vi "AbelFcsMain.vi"() -> ()   [LabVIEW 2011]
uses:
  <vilib>/vision/Pattern Matching.llb/IMAQ Curve Parameters.ctl
  <vilib>/vision/Pattern Matching.llb/IMAQ Match Range Setting.ctl
  Camera/lib/System Files/user.lib/atmcd32d.llb/Shutter_mode typedef.ctl
  Camera/lib/System Files/user.lib/atmcd32d.llb/Shutter_type typedef.ctl
  <vilib>/vision/Image Controls.llb/IMAQ Rounding Mode.ctl
  Variables/patternImg.vi
  Camera/vi/GlobalSetGetConfigureCamera.vi
  Camera/vi/ccdChipPixels.vi
  Variables/GetPicture.vi
  Variables/GlobalConAxisPI.vi
  Variables/GlobalLaserInterface.vi
  Camera/vi/StopGetPic.vi
  Camera/vi/CamDef.vi
panel:
  out "subarray":dbl[](array[numeric])
  in  "Settings (GeometricMatching)":T3={"Curve Parameters"={"Extraction Mode"=0, "Edge Threshold"=75, "Edge Filter Size"=1, "Min Length"=25, "Row Search Step Size"=15, "Col Search Step Size"=15, "Max Endpoint Gap"=10, "Closed"=FALSE, "Subpixel"=FALSE}, "Match Mode"={"Rotation"=TRUE, "Scale"=FALSE, "Occlusion"=TRUE, "Reserved"=FALSE, "Reserved"=FALSE, "Reserved"=FALSE}, "Range Settings"=[{"Match Constraints"=0, "Min"=0.0, "Max"=360.0}, {"Match Constraints"=2, "Min"=0.0, "Max"=25.0}], "Number of Matches"=5, "Minimum Match Score"=600.0, "SubPixel Accuracy"=FALSE, "Adv. Geometric Match Options 2"=[{"Setup Data Item"=21, "Item Value"=0.0}, {"Setup Data Item"=22, "Item Value"=1.0}]} {"Curve Parameters"."Extraction Mode" items=["Normal", "Uniform Regions"]; "Curve Parameters"."Edge Filter Size" items=["Fine", "Normal", "Contour Tracing"]; "Curve Parameters"."Max Endpoint Gap" min=0; "Curve Parameters"."Col Search Step Size" min=1 max=255 step=1; "Curve Parameters"."Row Search Step Size" min=1 max=255 step=1; "Curve Parameters"."Min Length" min=0; "Curve Parameters"."Edge Threshold" min=1 max=350 step=1; "Range Settings"."Max" format="%.2f"; "Range Settings"."Min" format="%.2f"; "Range Settings"."Match Constraints" items=["Rotation Angle (degrees)", "Scale Factor (%)", "Occlusion (%)"]; "Adv. Geometric Match Options 2"."Setup Data Item" items=["Curve Extraction Mode", "Curve Edge Threshold", "Curve Edge Filter Size", "Min Curve Length", "Curve Row Search Step Size", "Curve Col Search Step Size", "Curve Max Endpoint Gap", "Extract Closed Curves", "Enable Subpixel Curve Extraction", "Enable Correlation Score", "Enable Subpixel Accuracy", "Subpixel Iterations", "Subpixel Tolerance", "Initial Match List Length", "Enable Target Template Curve Score", "Min Match Separation Distance", "Min Match Separation Angle", "Min Match Separation Scale", "Max Match Overlap", "Enable Coarse Result", "Enable Calibration Support", "Enable Contrast Reversal", "Search Strategy", "Refinement Match Factor", "Subpixel Match Factor"]}
  in  "Tab Control":T4(tab)
  out "Histogram":i32[][](graph)
  out "Trace":i32[][](graph)=[[2, 0, 0, 1, 1, 1, 0, 0, 0, 1, 0, 1, 0, 1, 2, 2, 0, 3, 0, 2, 2, 1, 3, 1, 0, 1, 1, 1, 0, 1, 3, 1, 0, 2, 0, 1, 0, 1, 1, 0, 1, 1, 3, 1, 0, 2, 0, 1, 1, 0, 0, 2, 0, 0, 1, 1, 1, 0, 0, 1, 0, 1, 0, 0, 0, 1, 2, 1, 1, 2, 0, 2, 4, 3, 1, 1, 0, 0, 1, 1, 2, 0, 1, 1, 0, 0, 0, 1, 1, 1, 1, 3, 0, 0, 1, 0, 0, 0, 2, 1, 1, 1, 2, 1, 0, 1, 1, 0, 0, 2, 1, 1, 0, 0, 1, 1, 1, 1, 0, 2, 2, 0, 1, 2, 1, 0, 3, 0, 2, 1, 3, 0, 1, 1, 0, 0, 3, 0, 0, 0, 0, 0, 0, 0, 0, 0, 0, 0, 0, 0, 0, 0, 0, 0, 0, 0, 0, 0, 0, 0, 0, 0, 0, 0, 0, 0, 0, 0, 0, 0, 0, 0, 0, 0, 0, 0, 0, 0, 0, 0, 0, 0, 0, 0, 0, 0, 0, 0, 0, 0, 0, 0, 0, 0, 0, 0, 0, 0, 0, 0], [1, 2, 2, 0, 0, 0, 1, 2, 1, 2, 1, 1, 1, 0, 0, 0, 3, 1, 0, 1, 0, 2, 0, 2, 1, 1, 0, 0, 1, 0, 1, 2, 1, 0, 0, 0, 0, 0, 1, 0, 1, 0, 2, 0, 1, 0, 0, 0, 0, 1, 1, 3, 0, 0, 0, 2, 0, 0, 2, 0, 1, 1, 0, 0, 2, 0, 2, 1, 0, 1, 1, 0, 1, 1, 0, 0, 0, 1, 0, 0, 1, 0, 0, 0, 0, 1, 0, 1, 1, 1, 1, 0, 0, 0, 1, 1, 1, 0, 1, 0, 0, 0, 1, 1, 1, 0, 0, 1, 1, 3, 1, 0, 0, 0, 0, 0, 0, 0, 1, 2, 1, 0, 0, 0, 2, 3, 3, 2, 0, 1, 1, 1, 0, 0, 4, 0, 1, 2, 0, 0, 0, 2, 0, 0, 0, 0, 0, 0, 0, 0, 0, 0, 0, 0, 0, 0, 0, 0, 0, 0, 0, 0, 0, 0, 0, 0, 0, 0, 0, 0, 0, 0, 0, 0, 0, 0, 0, 0, 0, 0, 0, 0, 0, 0, 0, 0, 0, 0, 0, 0, 0, 0, 0, 0, 0, 0, 0, 0, 0, 0], [2, 2, 0, 1, 2, 0, 1, 0, 2, 3, 1, 0, 1, 0, 1, 0, 0, 0, 0, 2, 1, 0, 0, 2, 2, 0, 0, 0, 3, 0, 0, 2, 2, 2, 0, 3, 0, 3, 1, 3, 1, 3, 1, 0, 3, 1, 3, 3, 1, 1, 1, 1, 2, 0, 1, 0, 1, 1, 1, 3, 0, 2, 3, 1, 1, 1, 0, 1, 0, 1, 2, 3, 1, 2, 1, 3, 0, 2, 0, 2, 0, 1, 0, 2, 2, 1, 1, 3, 1, 2, 1, 1, 1, 3, 0, 0, 0, 0, 1, 1, 1, 0, 1, 0, 2, 1, 1, 0, 1, 0, 1, 2, 2, 2, 2, 0, 1, 0, 0, 0, 1, 1, 2, 0, 0, 1, 5, 2, 2, 0, 2, 0, 2, 2, 2, 0, 1, 0, 6, 0, 0, 0, 0, 0, 0, 0, 0, 0, 0, 0, 0, 0, 0, 0, 0, 0, 0, 0, 0, 0, 0, 0, 0, 0, 0, 0, 0, 0, 0, 0, 0, 0, 0, 0, 0, 0, 0, 0, 0, 0, 0, 0, 0, 0, 0, 0, 0, 0, 0, 0, 0, 0, 0, 0, 0, 0, 0, 0, 0, 0], [0, 0, 1, 0, 1, 1, 0, 0, 0, 1, 1, 0, 1, 0, 0, 0, 0, 0, 2, 0, 0, 0, 0, 2, 0, 0, 0, 1, 1, 2, 1, 1, 1, 2, 1, 0, 0, 3, 0, 1, 1, 0, 0, 0, 0, 1, 0, 0, 2, 1, 0, 0, 1, 1, 1, 2, 2, 0, 1, 0, 0, 1, 0, 1, 1, 0, 0, 2, 1, 1, 2, 1, 1, 0, 0, 0, 0, 2, 1, 0, 0, 0, 0, 1, 0, 1, 0, 0, 0, 0, 1, 0, 0, 0, 0, 1, 0, 1, 1, 1, 0, 2, 3, 1, 1, 0, 1, 1, 1, 0, 1, 0, 0, 1, 1, 0, 2, 0, 0, 0, 0, 3, 0, 0, 0, 0, 0, 0, 0, 0, 1, 0, 2, 0, 0, 0, 1, 2, 2, 0, 1, 0, 0, 0, 0, 0, 0, 0, 0, 0, 0, 0, 0, 0, 0, 0, 0, 0, 0, 0, 0, 0, 0, 0, 0, 0, 0, 0, 0, 0, 0, 0, 0, 0, 0, 0, 0, 0, 0, 0, 0, 0, 0, 0, 0, 0, 0, 0, 0, 0, 0, 0, 0, 0, 0, 0, 0, 0, 0, 0]]
  out "Point":dbl[][](graph)
  out "Image Out":T5(plugin-control)
  out "Image Number":u32
  out "acquired FPS":dbl
  out "Image":i32[][](graph)
  out "AM image":T5(plugin-control)
  out "Number of Particles":i32
  out "Image 2":dbl[][](graph)
  out "Auto Measure Points":i32
  out "NxtAutMesPoint":i32
  out "Pattern":dbl[][](array[numeric])
  out "X Steps":dbl
  out "3dAbelFcs":bool=TRUE
  out "Y Steps":dbl
  out "Z Steps":dbl
  out "concatenated string":string
  out "Global Stop":bool=TRUE
  out "Stop Measurement":bool
  in  "DeviceTabs":T6(tab)
  in  "WS File Tree":string(tree)
  out "Workspace":path=path "X:/MTusers/Christoph/2011-02-01 Andi/2011-02-01.msw"
  in  "New MSW":bool
  in  "Open MSW":bool
  in  "Sample description":string
  in  "Save Files":bool=TRUE
  out "Last Image File No":i32=-1
  in  "Get Position":bool
  in  "Move Stage":bool
  in  "X-Position":dbl=48.0021 caption="X" min=0.0 max=200.0 step=0.1 format="%1.3f um"
  in  "Y-Position":dbl=19.9997 caption="Y" min=0.0 max=200.0 step=0.1 format="%1.3f um"
  in  "Z-Position":dbl=69.999 caption="Z" min=0.0 max=200.0 step=0.1 format="%1.3f um"
  out "x-position":dbl format="%.3f"
  out "y-position":dbl format="%.3f"
  out "z-position":dbl format="%.3f"
  in  "CFD Settings":T7={"Sync Level"=17, "Sync ZeroX"=0, "Sync Offset"=0, "Chan Settings"=[{"CHx Level"=50, "CHx ZeroX"=10, "CHx Offset"=-22150}, {"CHx Level"=50, "CHx ZeroX"=10, "CHx Offset"=-21850}, {"CHx Level"=75, "CHx ZeroX"=10, "CHx Offset"=-6000}, {"CHx Level"=75, "CHx ZeroX"=10, "CHx Offset"=-5700}]}
  in  "Laser  Profile":string="1"
  in  "Auto Exposure::Mode":u32(ring) items=["Relative"=0, "Ignored"=5]
  in  "Brightness::Mode":u32(ring) items=["Relative"=0, "Ignored"=5]
  in  "Gain::Mode":u32(ring) items=["Absolute"=1, "Auto"=3, "Relative"=0, "Ignored"=5]
  in  "Gamma::Mode":u32(ring)=2 items=["Relative"=0, "Off"=2, "Ignored"=5]
  in  "Shutter::Mode":u32(ring) items=["Auto"=3, "Relative"=0, "Ignored"=5]
  in  "Trigger::Trigger Activation":u32(ring) items=["Level Low", "Level High"]
  in  "Trigger::Trigger Mode":u32(ring)=16 items=["Mode 0"=0, "Mode 1"=1, "Mode 15"=15, "Off"=16]
  in  "Trigger Delay::Mode":u32(ring)=2 items=["Absolute"=1, "Relative"=0, "Off"=2, "Ignored"=5]
  in  "Brightness::Value":dbl=16.0 min=0.0 max=1023.0 step=1.0
  in  "Shutter::Value":dbl=436.0 min=1.0 max=4095.0 step=1.0
  in  "Auto Exposure::Value":dbl=125.0 min=50.0 max=205.0 step=1.0
  in  "Gain::Value":dbl min=0.0 max=680.0 step=1.0
  in  "Trigger::Trigger Parameter":u32 max=0
  in  "Get Temperature":bool
  in  "SET CCD":bool
  in  "OPEN SHUTER":bool
  in  "Close":bool
  in  "Gain":bool
  in  "Start":bool
  in  "Stop":bool
  in  "Exposure":bool
  in  "Set Temperature":bool
  in  "duty cycle":dbl=0.5 format="%.6f"
  in  "frequency":dbl=1.0 format="%.6f"
  in  "PI SystemNumber":i32=1
  in  "Image Measurent Parameters":T8
  in  "Measurement Tab Control":T9(tab)
  in  "SCANNER EMERGENCY":bool
  in  "Stop Program":bool
  out "Task":T10(ring)
  in  "Point Defocussed Cam":bool
  in  "Adjustment":bool
  in  "Laser pulse duration":i32[](array[numeric]) min=2 max=100000 step=1 format="%d µs"
  in  "Measurement Time":i32=60 min=10 format="%.0d s"
  in  "Point Measurement":bool
  out "Counts":u32[](array[numeric])
  in  "Axis":enum32{"x-y", "x-z", "y-x", "y-z", "z-x", "z-y"}(ring)
  in  "Picture size 2":dbl=10.0 min=0.1 max=200.0 format="%1.1f um"
  in  "Picture size":dbl=10.0 min=0.1 max=200.0 format="%1.1f um"
  in  "Pixel time":dbl=3.0 min=0.1 max=100.0 step=0.1 format="%.1f ms"
  in  "Resolution":dbl=0.08 min=0.01 max=10.0 step=0.01 format="%.2f µm"
  out "Measure. time":dbl format="%7.1f s"
  in  "Aquire Image":bool
  out "y":i16=500
  out "x":i16=500
  in  "Save Color Image":bool
  in  "Cam (Defocused)":bool
  in  "How long?":bool
  out "Estimated Time (h)":dbl
  in  "Mesaurement Time (Sec) / Step":dbl
  in  "Start 3D FCS Abel Scan":bool
  in  "FCS Point Measurement":bool
  in  "Z Stepsize":dbl
  in  "Y Stepsize":dbl
  in  "X Stepsize":dbl
  in  "Z End":dbl
  in  "Y End":dbl
  in  "X End":dbl
  in  "Z Start":dbl
  in  "Y Start":dbl
  in  "X Start":dbl
  in  "Find Mols":bool
  in  "Filter":bool=TRUE
  in  "Remove Outliers":i32=10
  in  "Exclude / Include X":bool
  in  "X Start 2":dbl
  in  "X End 2":dbl
  in  "Exclude / Include Y":bool
  in  "Y Start 2":dbl
  in  "Y End 2":dbl
  in  "Measurement Parameter 1":T11 items=["Center of Mass X", "Center of Mass Y", "First Pixel X", "First Pixel Y", "Bounding Rect Left", "Bounding Rect Top", "Bounding Rect Right", "Bounding Rect Bottom", "Max Feret Diameter Start X", "Max Feret Diameter Start Y", "Max Feret Diameter End X", "Max Feret Diameter End Y", "Max Horiz. Segment Length Left", "Max Horiz. Segment Length Right", "Max Horiz. Segment Length Row", "-", "Bounding Rect Width", "Bounding Rect Height", "Bounding Rect Diagonal", "Perimeter", "Convex Hull Perimeter", "Holes' Perimeter", "Max Feret Diameter", "Equivalent Ellipse Major Axis", "Equivalent Ellipse Minor Axis", "Equivalent Ellipse Minor Axis (Feret)", "Equivalent Rect Long Side", "Equivalent Rect Short Side", "Equivalent Rect Diagonal", "Equivalent Rect Short Side (Feret)", "Average Horiz. Segment Length", "Average Vert. Segment Length", "Hydraulic Radius", "Waddel Disk Diameter", "-", "Area", "Holes' Area", "Particle & Holes' Area", "Convex Hull Area", "Image Area", "-", "Number of Holes", "Number of Horiz. Segments", "Number of Vert. Segments", "-", "Orientation", "Max Feret Diameter Orientation", "-", "% Area/Image Area", "% Area/(Particle & Holes' Area)", "Ratio of Equivalent Ellipse Axes", "Ratio of Equivalent Rect Sides", "-", "Elongation Factor", "Compactness Factor", "Heywood Circularity Factor", "Type Factor", "-", "Sum X", "Sum Y", "Sum XX", "Sum XY", "Sum YY", "Sum XXX", "Sum XXY", "Sum XYY", "Sum YYY", "-", "Moment of Inertia XX", "Moment of Inertia XY", "Moment of Inertia YY", "Moment of Inertia XXX", "Moment of Inertia XXY", "Moment of Inertia XYY", "Moment of Inertia YYY", "Norm. Moment of Inertia XX", "Norm. Moment of Inertia XY", "Norm. Moment of Inertia YY", "Norm. Moment of Inertia XXX", "Norm. Moment of Inertia XXY", "Norm. Moment of Inertia XYY", "Norm. Moment of Inertia YYY", "Hu Moment 1", "Hu Moment 2", "Hu Moment 3", "Hu Moment 4", "Hu Moment 5", "Hu Moment 6", "Hu Moment 7"]
  in  "Range Lower Value Par 1":dbl
  in  "Range Upper Value  Par 1":dbl
  in  "Ex/In Par 1":bool
  in  "Measurement Parameter 2":T11 items=["Center of Mass X", "Center of Mass Y", "First Pixel X", "First Pixel Y", "Bounding Rect Left", "Bounding Rect Top", "Bounding Rect Right", "Bounding Rect Bottom", "Max Feret Diameter Start X", "Max Feret Diameter Start Y", "Max Feret Diameter End X", "Max Feret Diameter End Y", "Max Horiz. Segment Length Left", "Max Horiz. Segment Length Right", "Max Horiz. Segment Length Row", "-", "Bounding Rect Width", "Bounding Rect Height", "Bounding Rect Diagonal", "Perimeter", "Convex Hull Perimeter", "Holes' Perimeter", "Max Feret Diameter", "Equivalent Ellipse Major Axis", "Equivalent Ellipse Minor Axis", "Equivalent Ellipse Minor Axis (Feret)", "Equivalent Rect Long Side", "Equivalent Rect Short Side", "Equivalent Rect Diagonal", "Equivalent Rect Short Side (Feret)", "Average Horiz. Segment Length", "Average Vert. Segment Length", "Hydraulic Radius", "Waddel Disk Diameter", "-", "Area", "Holes' Area", "Particle & Holes' Area", "Convex Hull Area", "Image Area", "-", "Number of Holes", "Number of Horiz. Segments", "Number of Vert. Segments", "-", "Orientation", "Max Feret Diameter Orientation", "-", "% Area/Image Area", "% Area/(Particle & Holes' Area)", "Ratio of Equivalent Ellipse Axes", "Ratio of Equivalent Rect Sides", "-", "Elongation Factor", "Compactness Factor", "Heywood Circularity Factor", "Type Factor", "-", "Sum X", "Sum Y", "Sum XX", "Sum XY", "Sum YY", "Sum XXX", "Sum XXY", "Sum XYY", "Sum YYY", "-", "Moment of Inertia XX", "Moment of Inertia XY", "Moment of Inertia YY", "Moment of Inertia XXX", "Moment of Inertia XXY", "Moment of Inertia XYY", "Moment of Inertia YYY", "Norm. Moment of Inertia XX", "Norm. Moment of Inertia XY", "Norm. Moment of Inertia YY", "Norm. Moment of Inertia XXX", "Norm. Moment of Inertia XXY", "Norm. Moment of Inertia XYY", "Norm. Moment of Inertia YYY", "Hu Moment 1", "Hu Moment 2", "Hu Moment 3", "Hu Moment 4", "Hu Moment 5", "Hu Moment 6", "Hu Moment 7"]
  in  "Range Lower Value Par 2":dbl
  in  "Range Upper Value Par 2":dbl
  in  "Ex/In Par 2":bool
  in  "Square/Hexa":bool=TRUE
  in  "Connectivity 4/8":bool
  in  "Manual":bool
  in  "Focuswidth":dbl
  in  "Mode":enum16{"Gauss", "Radial", "Azimuthal"}(ring)
  in  "Detection Modus":u16(ring) items=["Pattern", "Heuristic"]
  in  "NA":dbl
  in  "Auto Defocussed Cam":bool
  in  "Autopoint-Autofocus Z":bool=TRUE
  in  "Auto Measurement Time (ms)":i32=60 caption="Measurement Time (s)" min=10
  out "Auto Meas Progress":i32(slide) caption="Point 34 / 34" scale=0.0..34.0
  in  "Auto Meas":bool
  out "Active pt3":path
  out "Buffer Overrun":bool
  out "Running":bool
  # "Range"
  # "Scanner Position"
  # "Point Measurement Settings"
  # "Start Experiment"
  # "Estimated Mesaurement Time"
  # "Image Scan Settings"
  # "Save as png"
  # "Pixel"
  # "Define the 3D Space and Stepwith of your Experiment"
  # "Time of the Experiment"
  # "Check What to Mesaure"
  # "Start Your Experiment here"
  # "Lifetime Mesaurement Time on each Position"
  # "Define Search Area"
  # "Define Detection Parameters"
  # "Exact Matching"
  # "Operation"
  # "Show Progress"
  # "Automated Mesaurement on Single Molecule Coordinates on the  2D Frame"
  # "Start Your Experiment here"
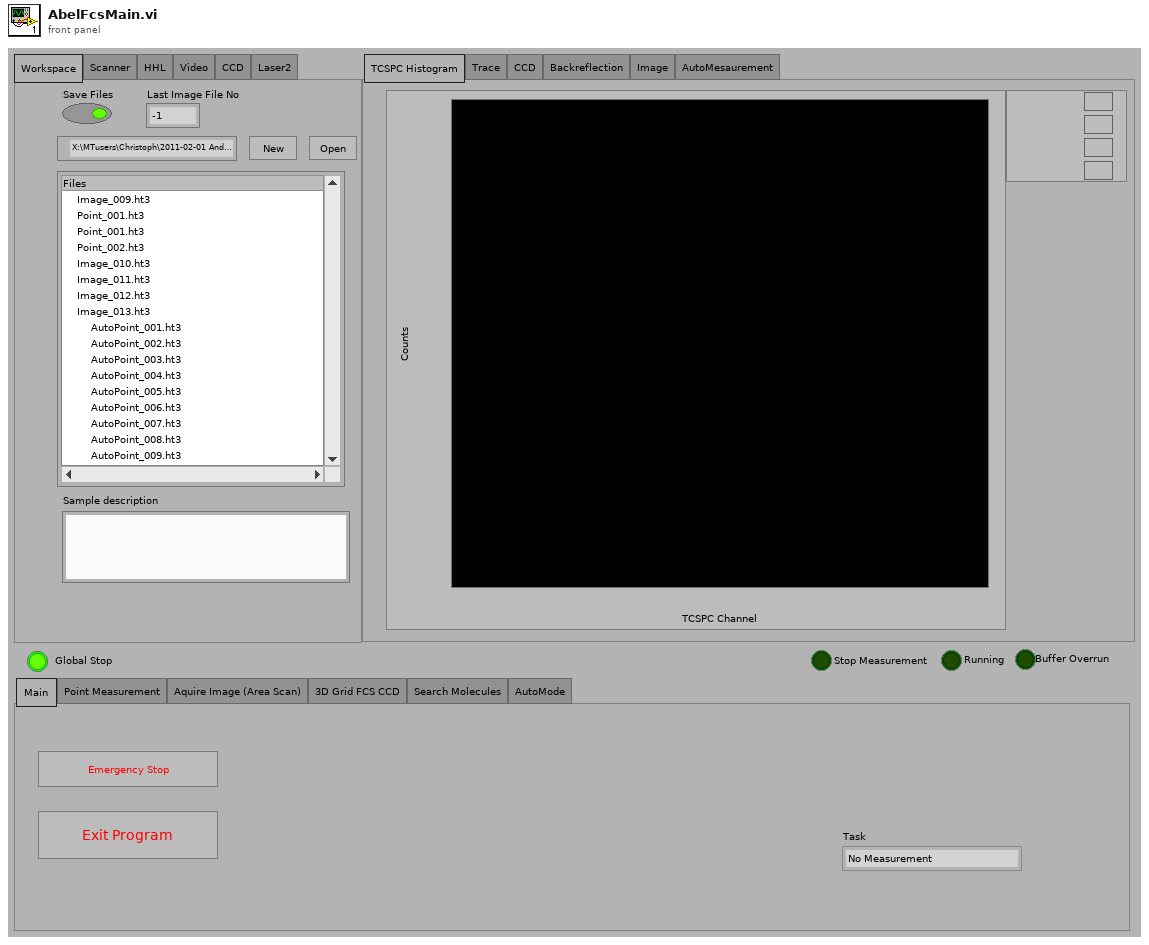
[diagram p1: front panel]
types:
  T1 = typedef "IMAQ Curve Parameters.ctl" = cluster{"Extraction Mode":u32, "Edge Threshold":i32, "Edge Filter Size":u32, "Min Length":i32, "Row Search Step Size":i32, "Col Search Step Size":i32, "Max Endpoint Gap":i32, "Closed":bool, "Subpixel":bool}
  T2 = typedef "IMAQ Match Range Setting.ctl" = cluster{"Match Constraints":u32, "Min":dbl, "Max":dbl}
  T3 = cluster{"Curve Parameters":T1, "Match Mode":cluster{"Rotation":bool, "Scale":bool, "Occlusion":bool, "Reserved":bool, "Reserved":bool, "Reserved":bool}, "Range Settings":T2[], "Number of Matches":i32, "Minimum Match Score":sgl, "SubPixel Accuracy":bool, "Adv. Geometric Match Options 2":cluster{"Setup Data Item":u16, "Item Value":dbl}[]}
  T4 = enum32{"TCSPC Histogram", "Trace", "CCD", "Backreflection", "Image", "AutoMesaurement"}
  T5 = typedef "IMAQ Image.ctl" = refnum<image>
  T6 = enum32{"Workspace", "Scanner", "HHL", "Video", "CCD", "Laser2"}
  T7 = cluster{"Sync Level":i32, "Sync ZeroX":i32, "Sync Offset":i32, "Chan Settings":cluster{"CHx Level":i32, "CHx ZeroX":i32, "CHx Offset":i32}[]}
  T8 = cluster{"Position":cluster{"X-Position":dbl, "Y-Position":dbl, "Z-Position":dbl}, "Axis 1 Pixels":dbl, "Axis 2 Pixels":dbl, "Axis":i32, "Resolution":dbl, "PixelTime":dbl, "Laser pulses":i32}
  T9 = enum32{"Main ", "Point Measurement", "Aquire Image (Area Scan)", "3D Grid FCS CCD", "Search Molecules", "AutoMode"}
  T10 = enum16{"No Measurement", "Aquire Image", "Point Measurement", "Multi Measurement", "Save Color Image", "Find Single Mol.", "Auto Measurement Control", "Auto Point", "Aquire Line Scan", "Grid Measurement", "Trapping", "Move Scanner"}
  T11 = typedef "Particle Parameters" = i32
  T12 = cluster{"Dev":i32, "SerNo":string, "HW_Model":string, "HW_Partno":string}[]
  T13 = enum16{"No Measurement", "Aquire Image", "Point Measurement", "Multi Measurement", "Save Color Image"}
  T14 = enum16{"No Measurement", "Aquire Image", "Point Measurement", "Multi Measurement", "Save Color Image", "Find Single Mol.", "Auto Measurement Control", "Auto Point"}
  T15 = enum16{"No Measurement", "Aquire Image", "Point Measurement", "Multi Measurement", "Save Color Image", "Find Single Mol."}
  T16 = enum16{"Get (Default)", "Set Workspace", "Append File", "Change Comment"}
  T17 = typedef "Shutter_type typedef.ctl" = enum16{"TTL Low", "TTL High"}
  T18 = typedef "Shutter_mode typedef.ctl" = enum16{"Auto", "Open", "Close"}
  T19 = cluster{"File No":i32, "File Path":path, "Parent File":i32, "File Type":enum16{"unknown", "pt3 File", "png Image", "bmp Image"}, "Measurement Type":enum16{"not a pt3 File", "Image File", "Point Measurement", "Auto Point", "Line Scan", "Grid Scan"}, "Upper Left":cluster{"x-Position":dbl, "y-Position":dbl, "z-Position":dbl}, "Pixels":dbl[], "Resolution":dbl, "Scan Axis":enum32{"x-y", "x-z", "y-x", "y-z", "z-x", "z-y"}, "PixelTime":dbl}[]
  T20 = cluster{"File No":i32, "File Path":path, "Parent File":i32, "File Type":enum16{"unknown", "pt3 File", "png Image", "bmp Image"}, "Measurement Type":enum16{"not a pt3 File", "Image File", "Point Measurement", "Auto Point", "Line Scan", "Grid Scan"}, "Upper Left":cluster{"x-Position":dbl, "y-Position":dbl, "z-Position":dbl}, "Pixels":i32[], "Scan Axis":enum32{"x-y", "x-z", "y-x", "y-z", "z-x", "z-y"}, "Resolution":dbl, "PixelTime":dbl}[]
  T21 = cluster{"File No":i32, "File Path":path, "Parent File":i32, "File Type":enum16{"unknown", "pt3 File", "png Image", "bmp Image"}, "Measurement Type":enum16{"not a pt3 File", "Image File", "Point Measurement", "Auto Point", "Line Scan", "Grid Scan"}, "Upper Left":cluster{"x-Position":dbl, "y-Position":dbl, "z-Position":dbl}, "Pixels":i32[], "Resolution":dbl, "Scan Axis":enum32{"x-y", "x-z", "y-z"}, "PixelTime":dbl}[]
  T22 = cluster{"Files in Workspace[0]":cluster{"File No":i32, "File Path":path, "Parent File":i32, "File Type":enum16{"unknown", "pt3 File", "png Image", "bmp Image"}, "Measurement Type":enum16{"not a pt3 File", "Image File", "Point Measurement", "Auto Point", "Line Scan", "Grid Scan"}, "Upper Left":cluster{"x-Position":dbl, "y-Position":dbl, "z-Position":dbl}, "Pixels":i32[], "Scan Axis":enum32{"x-y", "x-z", "y-x", "y-z", "z-x", "z-y"}, "Resolution":dbl, "PixelTime":dbl}, "Files in Workspace[1]":cluster{"File No":i32, "File Path":path, "Parent File":i32, "File Type":enum16{"unknown", "pt3 File", "png Image", "bmp Image"}, "Measurement Type":enum16{"not a pt3 File", "Image File", "Point Measurement", "Auto Point", "Line Scan", "Grid Scan"}, "Upper Left":cluster{"x-Position":dbl, "y-Position":dbl, "z-Position":dbl}, "Pixels":i32[], "Scan Axis":enum32{"x-y", "x-z", "y-x", "y-z", "z-x", "z-y"}, "Resolution":dbl, "PixelTime":dbl}, "Files in Workspace[2]":cluster{"File No":i32, "File Path":path, "Parent File":i32, "File Type":enum16{"unknown", "pt3 File", "png Image", "bmp Image"}, "Measurement Type":enum16{"not a pt3 File", "Image File", "Point Measurement", "Auto Point", "Line Scan", "Grid Scan"}, "Upper Left":cluster{"x-Position":dbl, "y-Position":dbl, "z-Position":dbl}, "Pixels":i32[], "Scan Axis":enum32{"x-y", "x-z", "y-x", "y-z", "z-x", "z-y"}, "Resolution":dbl, "PixelTime":dbl}, "Files in Workspace[3]":cluster{"File No":i32, "File Path":path, "Parent File":i32, "File Type":enum16{"unknown", "pt3 File", "png Image", "bmp Image"}, "Measurement Type":enum16{"not a pt3 File", "Image File", "Point Measurement", "Auto Point", "Line Scan", "Grid Scan"}, "Upper Left":cluster{"x-Position":dbl, "y-Position":dbl, "z-Position":dbl}, "Pixels":i32[], "Scan Axis":enum32{"x-y", "x-z", "y-x", "y-z", "z-x", "z-y"}, "Resolution":dbl, "PixelTime":dbl}, "Files in Workspace[4]":cluster{"File No":i32, "File Path":path, "Parent File":i32, "File Type":enum16{"unknown", "pt3 File", "png Image", "bmp Image"}, "Measurement Type":enum16{"not a pt3 File", "Image File", "Point Measurement", "Auto Point", "Line Scan", "Grid Scan"}, "Upper Left":cluster{"x-Position":dbl, "y-Position":dbl, "z-Position":dbl}, "Pixels":i32[], "Scan Axis":enum32{"x-y", "x-z", "y-x", "y-z", "z-x", "z-y"}, "Resolution":dbl, "PixelTime":dbl}, "Files in Workspace[5]":cluster{"File No":i32, "File Path":path, "Parent File":i32, "File Type":enum16{"unknown", "pt3 File", "png Image", "bmp Image"}, "Measurement Type":enum16{"not a pt3 File", "Image File", "Point Measurement", "Auto Point", "Line Scan", "Grid Scan"}, "Upper Left":cluster{"x-Position":dbl, "y-Position":dbl, "z-Position":dbl}, "Pixels":i32[], "Scan Axis":enum32{"x-y", "x-z", "y-x", "y-z", "z-x", "z-y"}, "Resolution":dbl, "PixelTime":dbl}, "Files in Workspace[6]":cluster{"File No":i32, "File Path":path, "Parent File":i32, "File Type":enum16{"unknown", "pt3 File", "png Image", "bmp Image"}, "Measurement Type":enum16{"not a pt3 File", "Image File", "Point Measurement", "Auto Point", "Line Scan", "Grid Scan"}, "Upper Left":cluster{"x-Position":dbl, "y-Position":dbl, "z-Position":dbl}, "Pixels":i32[], "Scan Axis":enum32{"x-y", "x-z", "y-x", "y-z", "z-x", "z-y"}, "Resolution":dbl, "PixelTime":dbl}, "Files in Workspace[7]":cluster{"File No":i32, "File Path":path, "Parent File":i32, "File Type":enum16{"unknown", "pt3 File", "png Image", "bmp Image"}, "Measurement Type":enum16{"not a pt3 File", "Image File", "Point Measurement", "Auto Point", "Line Scan", "Grid Scan"}, "Upper Left":cluster{"x-Position":dbl, "y-Position":dbl, "z-Position":dbl}, "Pixels":i32[], "Scan Axis":enum32{"x-y", "x-z", "y-x", "y-z", "z-x", "z-y"}, "Resolution":dbl, "PixelTime":dbl}, "Files in Workspace[8]":cluster{"File No":i32, "File Path":path, "Parent File":i32, "File Type":enum16{"unknown", "pt3 File", "png Image", "bmp Image"}, "Measurement Type":enum16{"not a pt3 File", "Image File", "Point Measurement", "Auto Point", "Line Scan", "Grid Scan"}, "Upper Left":cluster{"x-Position":dbl, "y-Position":dbl, "z-Position":dbl}, "Pixels":i32[], "Scan Axis":enum32{"x-y", "x-z", "y-x", "y-z", "z-x", "z-y"}, "Resolution":dbl, "PixelTime":dbl}}
  T23 = typedef "LVPoint32TypeDef.ctl" = cluster{"Horizontal":i32, "Vertical":i32}
  T24 = cluster{"Shift":bool, "Ctrl":bool, "Alt":bool, "Cmd":bool, "Opt":bool}
  T25 = enum16{"No Measurement", "Aquire Image", "Point Measurement", "Multi Measurement", "Save Color Image", "Find Single Mol.", "Auto Measurement Control", "Auto Point", "Aquire Line Scan", "Grid Measurement"}
  T26 = enum16{"none", "fast axis", "slow axis", "both axis", ""}
  T27 = enum16{"none", "fast axis", "slow axis", "both", ""}
  T28 = enum16{"target position", "relative position", "actual position", "position error"}
  T29 = enum16{"not a pt3 File", "Image File", "Point Measurement", "Auto Point"}
  T30 = enum16{"unknown", "pt3 File", "png Image", "bmp Image"}
  T31 = typedef "IMAQ Rounding Mode.ctl" = enum16{"Optimize", "Truncate"}
  T32 = cluster{"Measurement Parameter":T11, "Range Lower Value":dbl, "Range Upper Value":dbl, "Range":bool, "Measurement Type":bool}[]
  T33 = enum16{"not a pt3 File", "Image File", "Point Measurement", "Auto Point", "Line Scan"}
  T34 = cluster{"Dev":i32, "SerNo":string, "HW_Model":string, "HW_Partno":string}
  T35 = cluster{"Comment":string, "Binning":i32, "Offset":i32, "AcquisitionTime (ms)":i32, "HardwareSerial":i32, "SyncDivider":i32, "Resolution (ps)":dbl, "CFD Settings":cluster{"Sync Level":i32, "Sync ZeroX":i32, "Sync Offset":i32, "Chan Settings":cluster{"CHx Level":i32, "CHx ZeroX":i32, "CHx Offset":i32}[]}, "ModuleInfo":cluster{"modelcode":i32, "versioncode":i32}[], "BaseResolution (ps)":dbl, "RefClockSource":i32, "ChanInfo":cluster{"CHx Level":i32, "CHx ZeroX":i32, "CHx Offset":i32, "CHx modidx":i32}[], "SyncRate":i32, "InputsEnabled":i64}
  T36 = cluster{"Dimensions":i32, "Time Per Pixel [ms]":dbl, "Acceleration":i32, "Pattern":i32, "X0":sgl, "Y0":sgl, "Z0":dbl, "PixX":i32, "PixY":i32, "PixResol":sgl, "TStartTo":sgl, "TStoptTo":sgl, "TStartFro":sgl, "TStopFro":sgl}
  T37 = cluster{"InpRateFilePos":i64, "StopAfterFilePos":i64}
  T38 = cluster{"X-Position":dbl, "Y-Position":dbl, "Z-Position":dbl}
  T39 = cluster{"File No":i32, "File Path":path, "Parent File":i32, "File Type":enum16{"unknown", "pt3 File", "png Image", "bmp Image"}, "Measurement Type":enum16{"not a pt3 File", "Image File", "Point Measurement", "Auto Point", "Line Scan", "Grid Scan"}, "Upper Left":cluster{"x-Position":dbl, "y-Position":dbl, "z-Position":dbl}, "Pixels":i32[], "Scan Axis":enum32{"x-y", "x-z", "y-z"}, "Resolution":dbl, "PixelTime":dbl}
  T40 = enum16{"not a pt3 File", "Image File", "Point Measurement", "Auto Point", "Line Scan", "Grid Scan"}
  T41 = cluster{"Ident":string, "Format Version":string, "Creator Name":string, "Creator Version":string, "File Time":string, "Comment":string, "Laser":i32, "Binning":i32, "Offset":i32, "AcquisitionTime (ms)":i32, "HardwareSerial":i32, "SyncDivider":i32, "Resolution (ps)":dbl, "Rates":dbl[], "SyncRate":dbl, "CFD Settings":cluster{"Sync Level":i32, "Sync ZeroX":i32, "Sync Offset":i32, "Chan Settings":cluster{"CHx Level":i32, "CHx ZeroX":i32, "CHx Offset":i32}[]}}
  T42 = cluster{"x-Position":dbl, "y-Position":dbl, "z-Position":dbl}
  T43 = typedef "Image Type" = u32
  T44 = cluster{"MesaurementSelection[0]":cluster{"Measurement Parameter":T11, "Range Lower Value":dbl, "Range Upper Value":dbl, "Range":bool, "Measurement Type":bool}, "MesaurementSelection[1]":cluster{"Measurement Parameter":T11, "Range Lower Value":dbl, "Range Upper Value":dbl, "Range":bool, "Measurement Type":bool}, "MesaurementSelection[2]":cluster{"Measurement Parameter":T11, "Range Lower Value":dbl, "Range Upper Value":dbl, "Range":bool, "Measurement Type":bool}, "MesaurementSelection[3]":cluster{"Measurement Parameter":T11, "Range Lower Value":dbl, "Range Upper Value":dbl, "Range":bool, "Measurement Type":bool}, "MesaurementSelection[4]":cluster{"Measurement Parameter":T11, "Range Lower Value":dbl, "Range Upper Value":dbl, "Range":bool, "Measurement Type":bool}, "MesaurementSelection[5]":cluster{"Measurement Parameter":T11, "Range Lower Value":dbl, "Range Upper Value":dbl, "Range":bool, "Measurement Type":bool}, "MesaurementSelection[6]":cluster{"Measurement Parameter":T11, "Range Lower Value":dbl, "Range Upper Value":dbl, "Range":bool, "Measurement Type":bool}, "MesaurementSelection[7]":cluster{"Measurement Parameter":T11, "Range Lower Value":dbl, "Range Upper Value":dbl, "Range":bool, "Measurement Type":bool}, "MesaurementSelection[8]":cluster{"Measurement Parameter":T11, "Range Lower Value":dbl, "Range Upper Value":dbl, "Range":bool, "Measurement Type":bool}}
  T45 = cluster{"Measurement Parameter":T11, "Range Lower Value":dbl, "Range Upper Value":dbl, "Range":bool, "Measurement Type":bool}
  T46 = typedef "IMAQ Point" = cluster{"X":sgl, "Y":sgl}
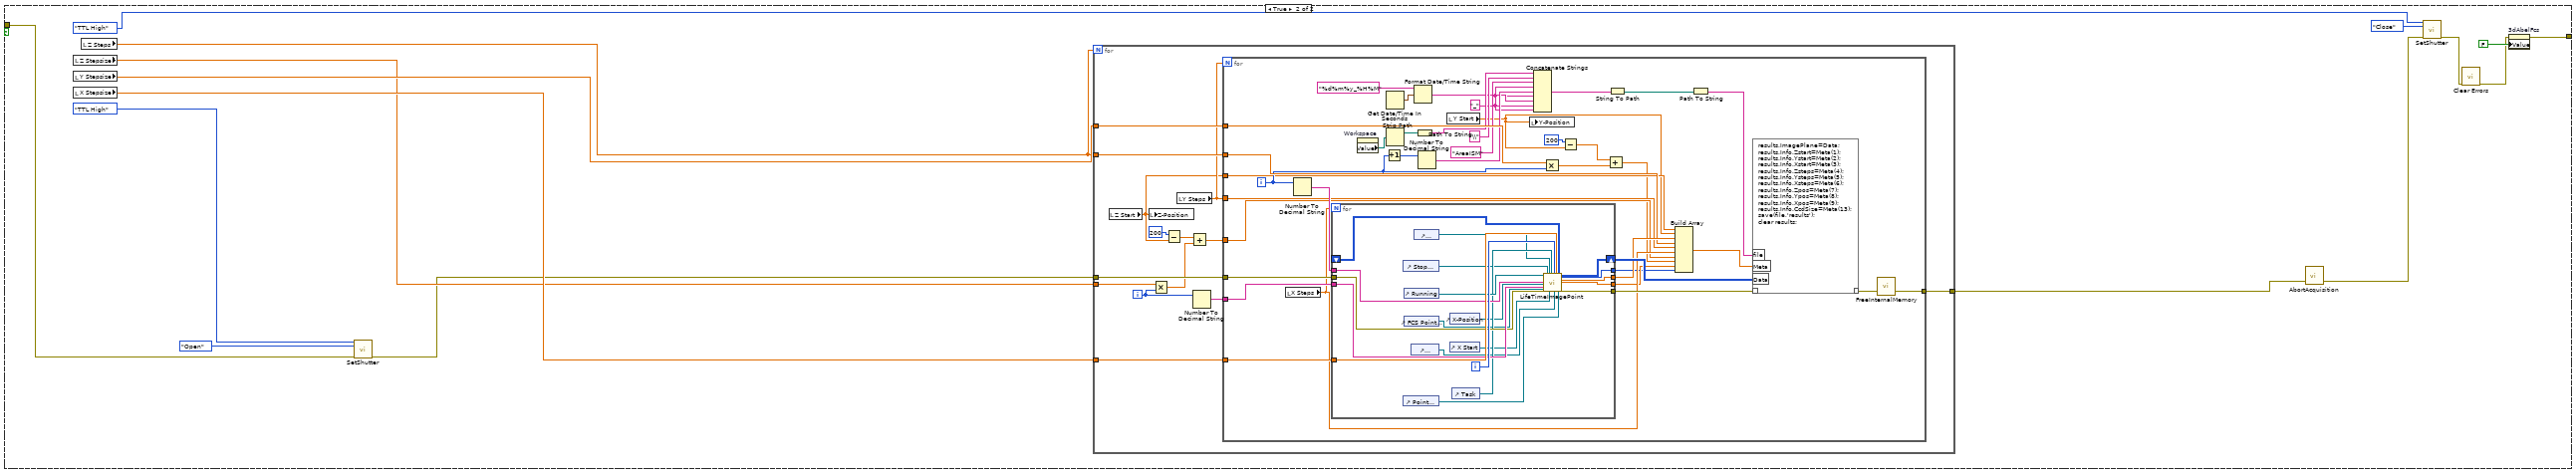
[diagram p2: hidden frame]
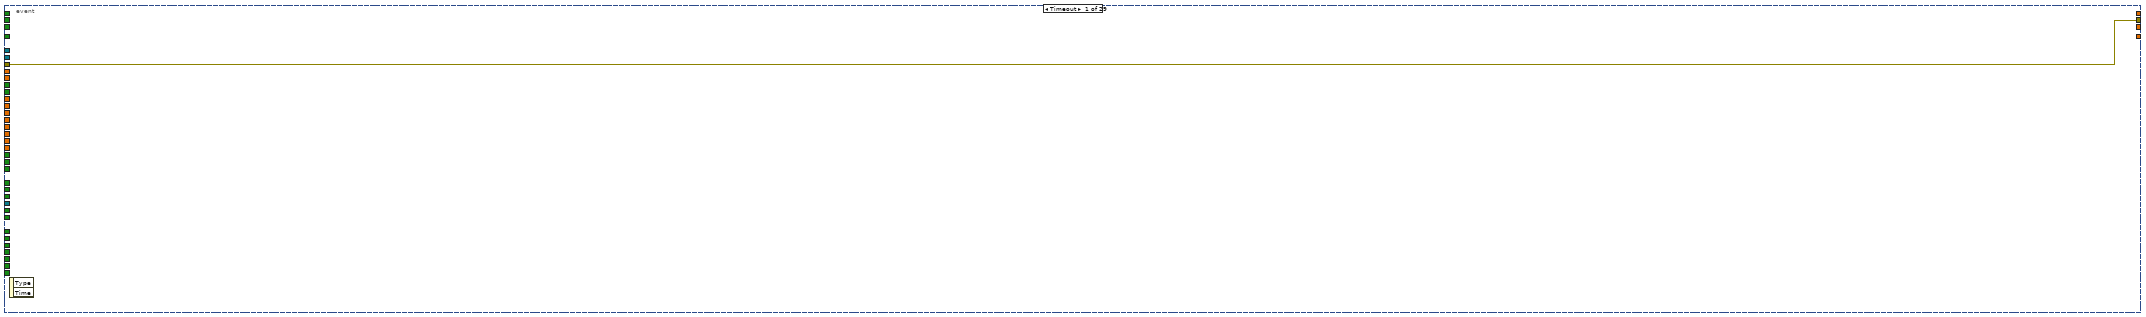
[diagram p3: hidden frame]
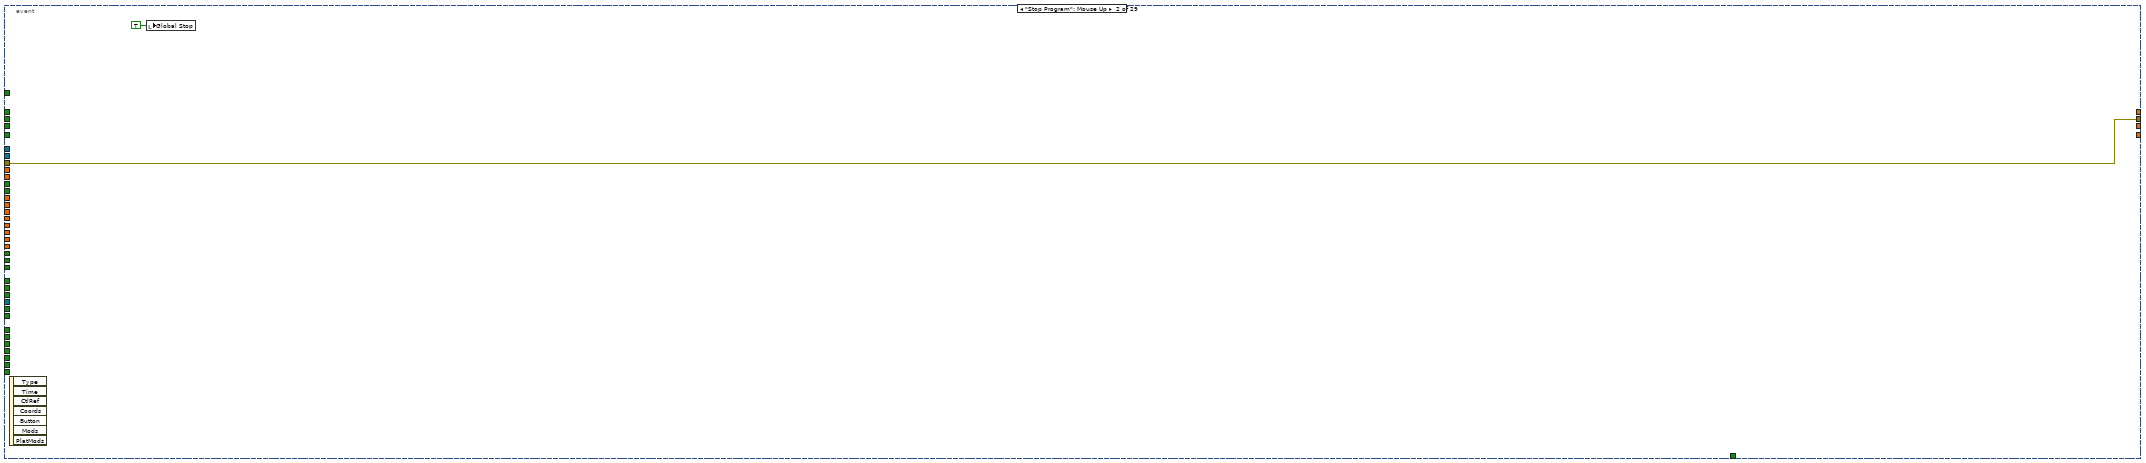
[diagram p4: hidden frame]
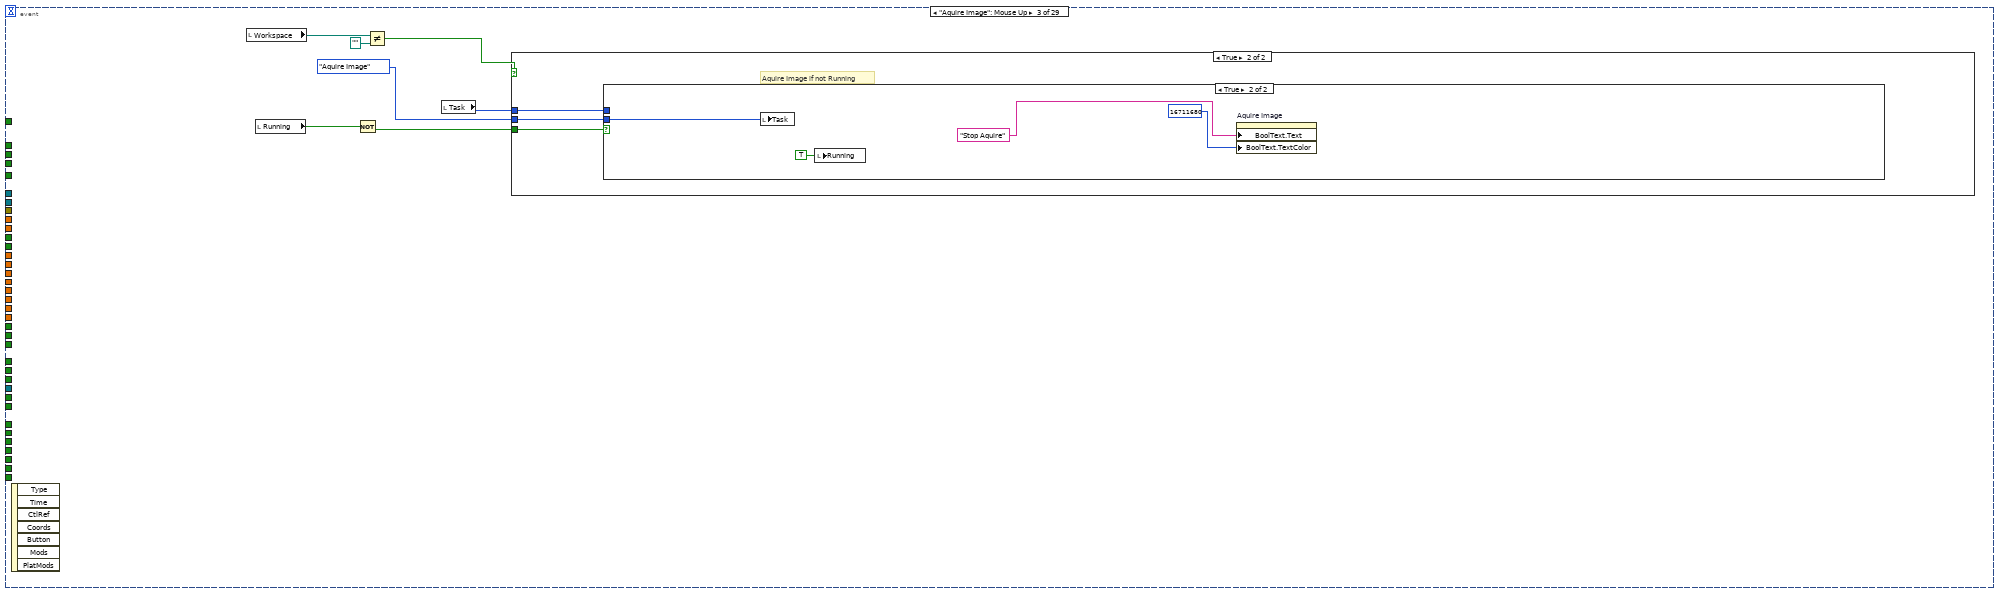
[diagram p5: hidden frame]
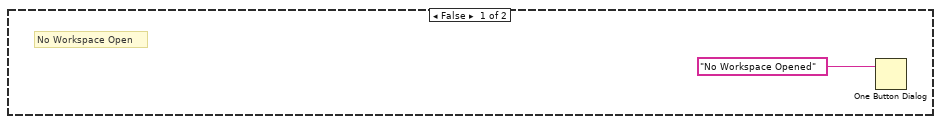
[diagram p6: hidden frame]
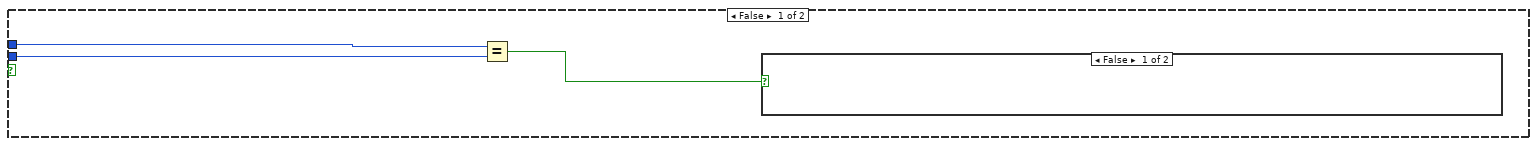
[diagram p7: hidden frame]
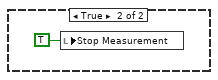
[diagram p8: hidden frame]
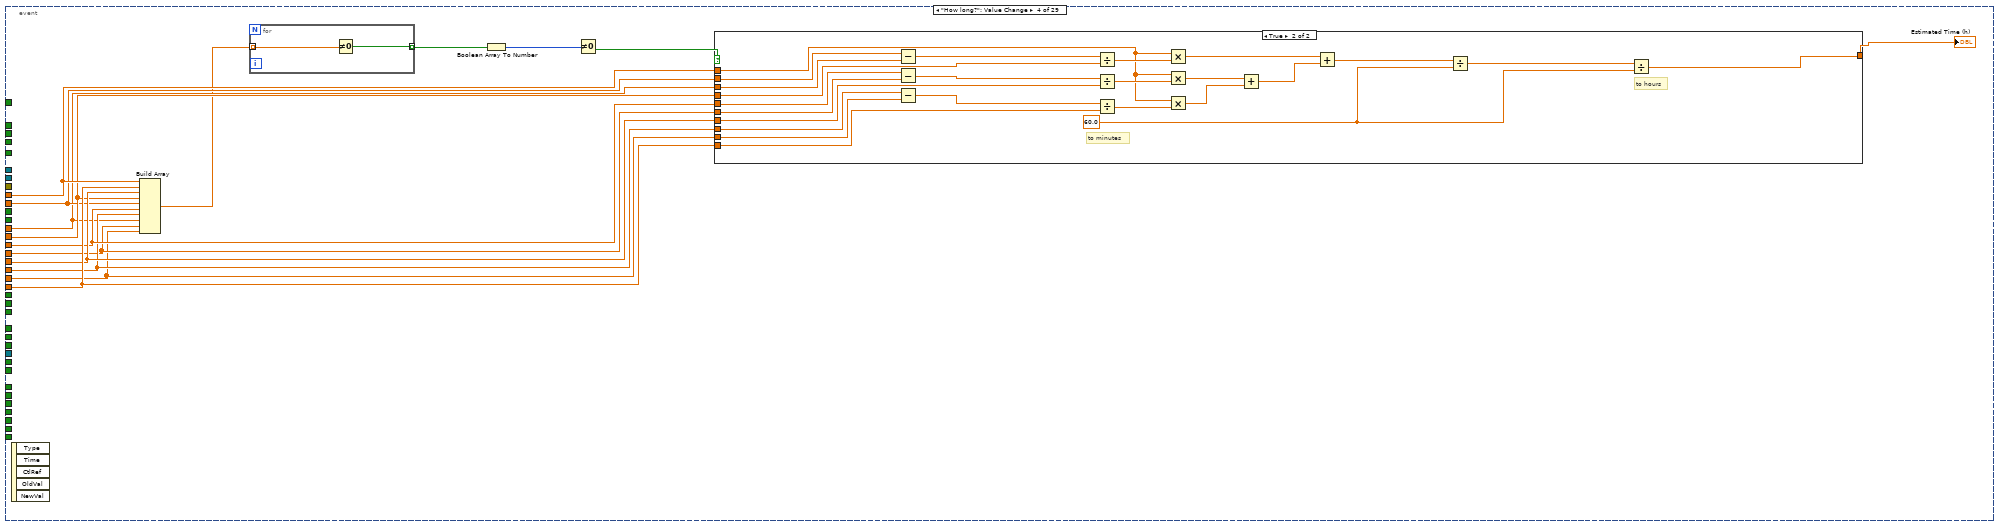
[diagram p9: hidden frame]
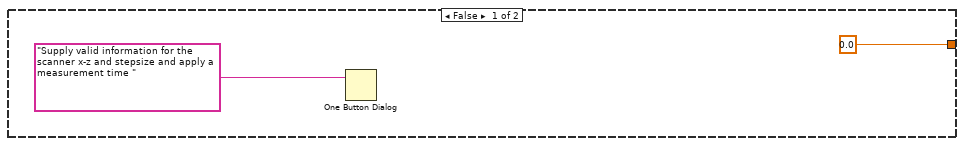
[diagram p10: hidden frame]
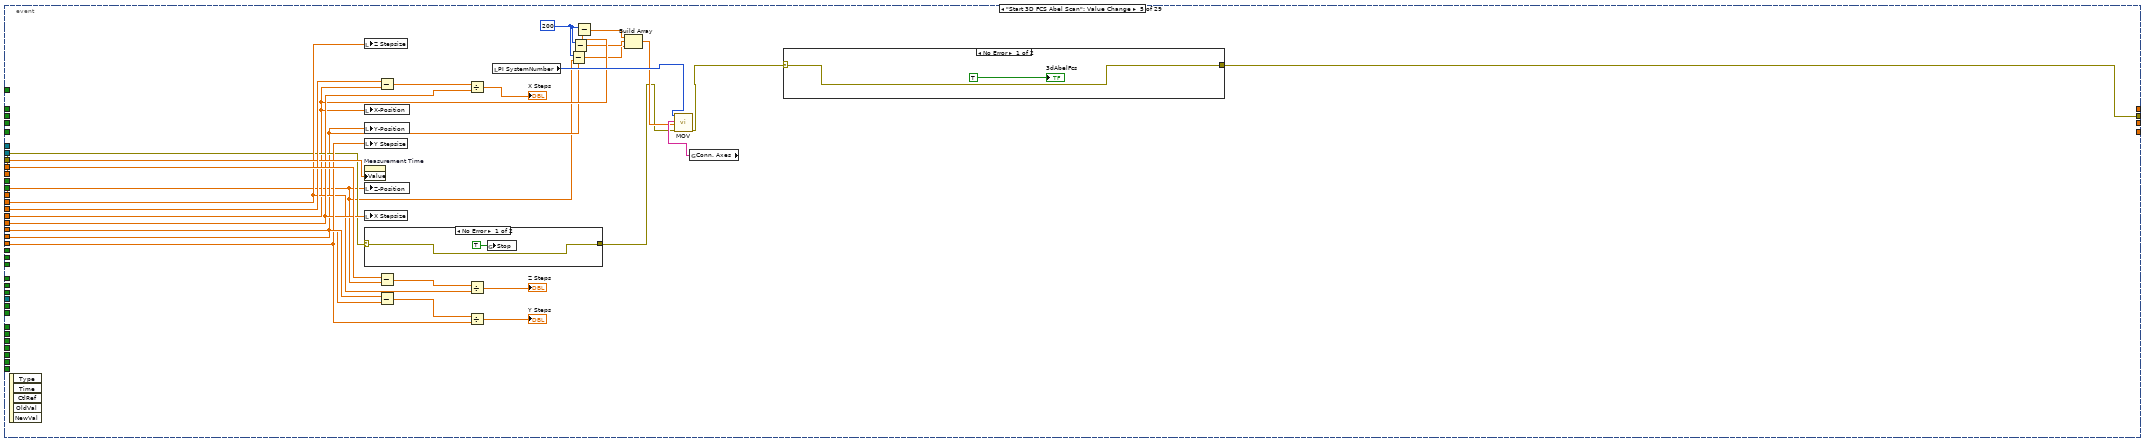
[diagram p11: hidden frame]
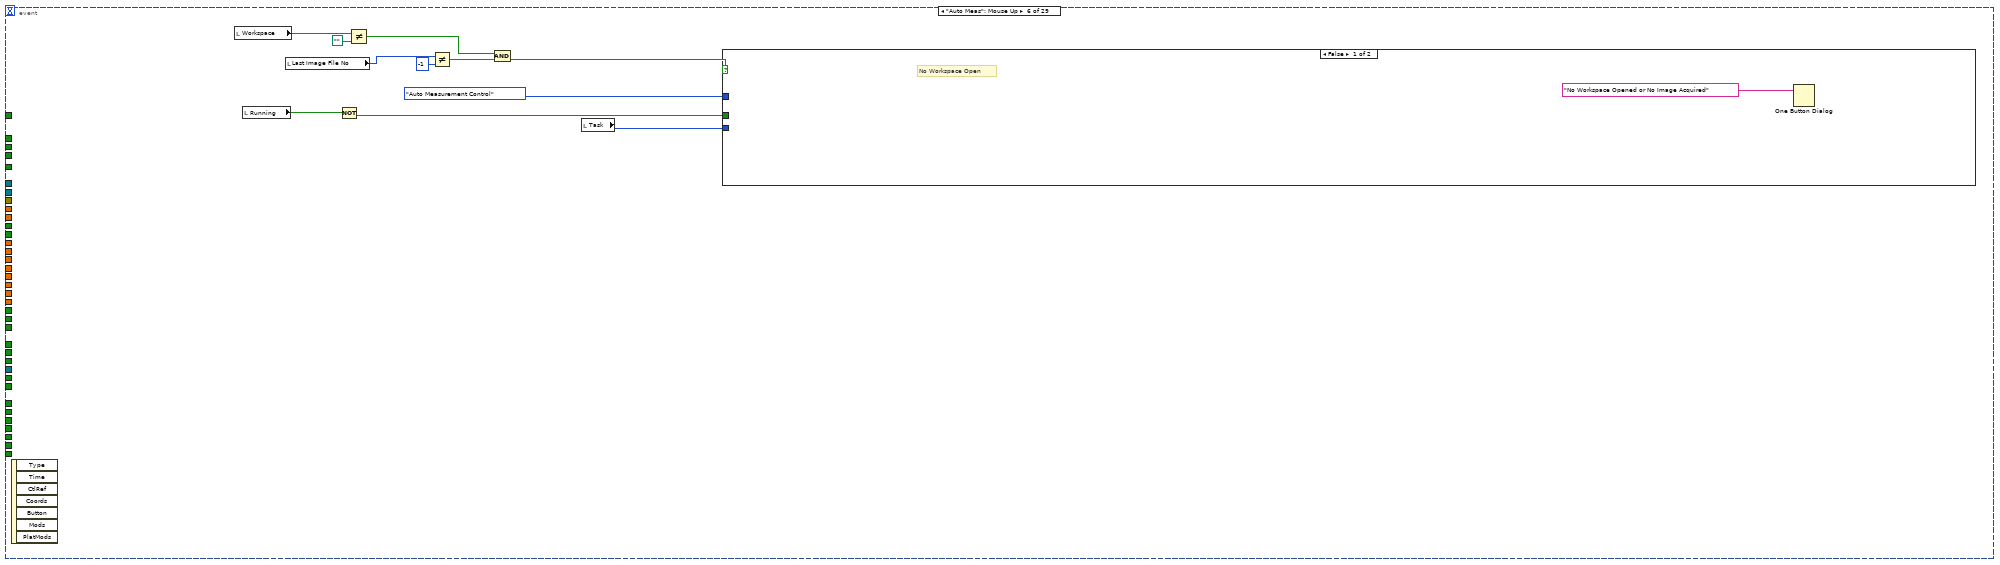
[diagram p14: hidden frame]
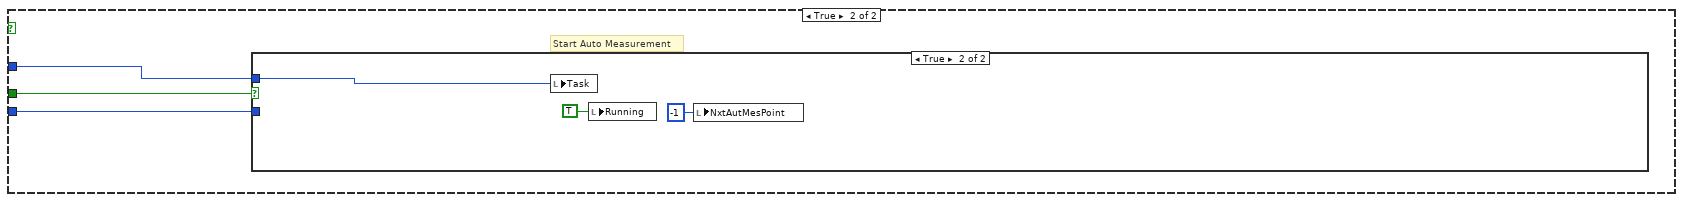
[diagram p15: hidden frame]
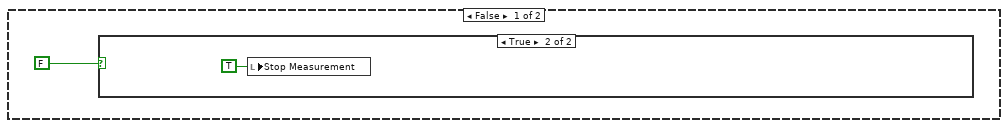
[diagram p16: hidden frame]
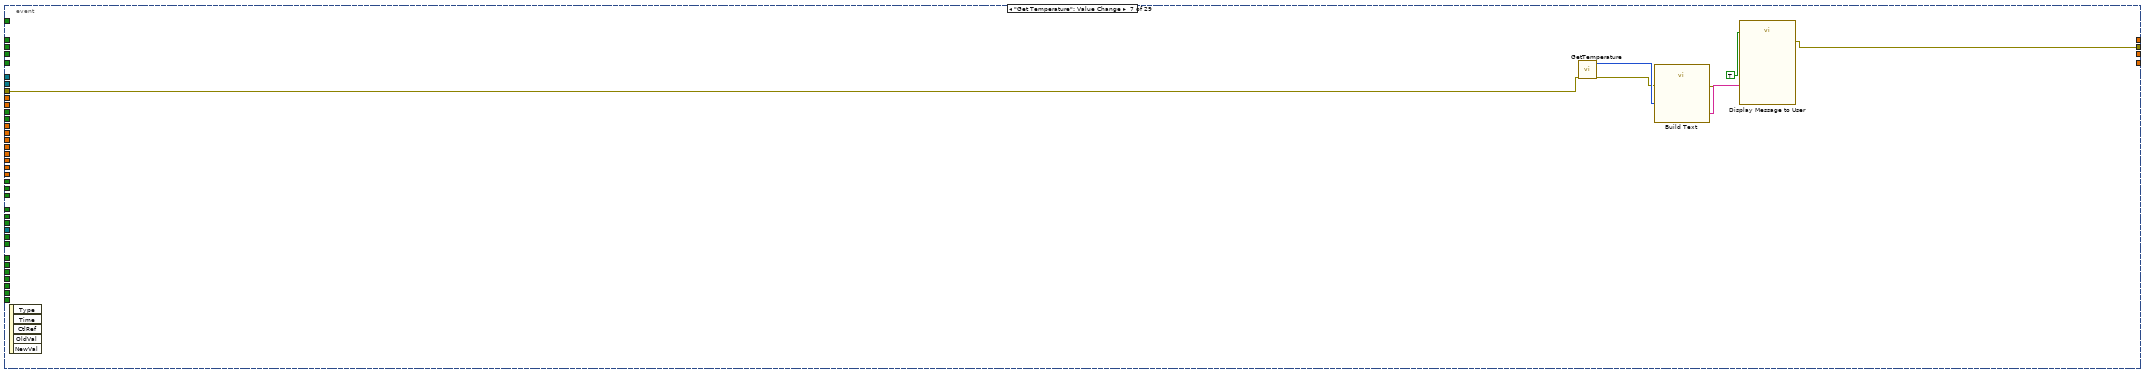
[diagram p18: hidden frame]
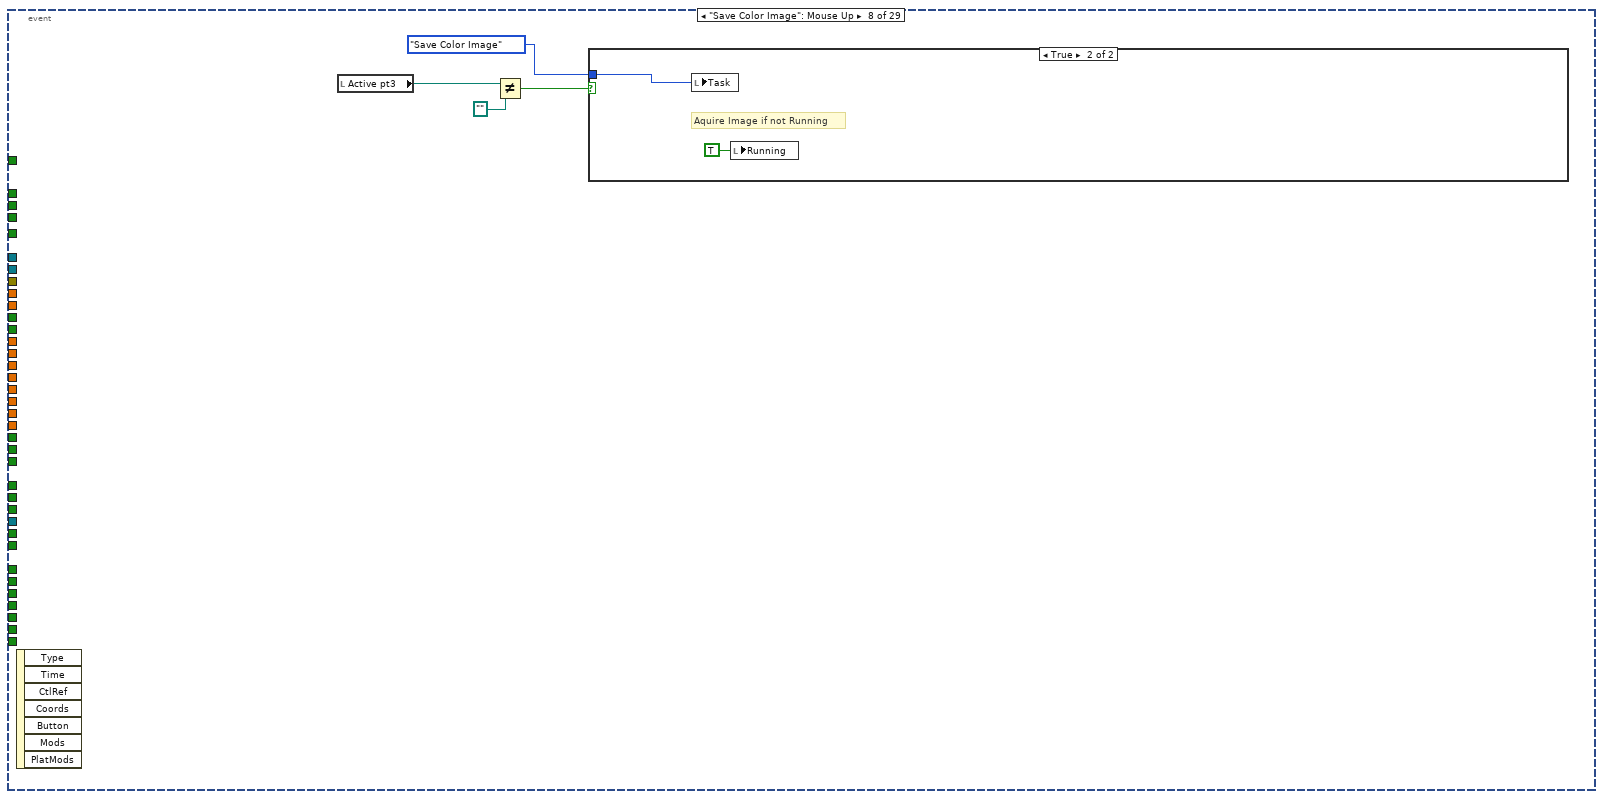
[diagram p19: hidden frame]
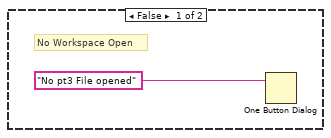
[diagram p20: hidden frame]
diagram:
  n1 = flat-sequence {
    tunnel: [w20] -> w14
    tunnel: errorcluster {"status"=FALSE, "code"=0, "source"=""} ("error in") -> [w31]
    frame #0 {
      (unwired) 1.0 ("CCD Chip Vertical Start")
      w32 = path ""
      w39 = FALSE ("Global Stop")
      n2 = control-ref of="WS File Tree"() -> (w38:refnum<vi>)
      n3 = global write "GetPicture.vi" "GetPicture"(FALSE ("GetPicture")) -> ()
      n4 = local write "Last Image File No"(-1 ("Last Image File No")) -> ()
      n5 = global write "GlobalSetGetConfigureCamera.vi" "gain"(30 ("gain")) -> ()
      n6 = global write "GlobalSetGetConfigureCamera.vi" "Exposure"(sgl 0.1 ("Exposure")) -> ()
      n7 = flat-sequence {
        tunnel: 1.0 ("Vertical Binning") -> [w45]
        tunnel: 1.0 ("CCD Chip Horizontal Start") -> [w44]
        tunnel: 1.0 ("CCD Chip Vertical Start") -> [w40]
        tunnel: 10.0 ("CCD Chip Horizontal End") -> [w43]
        tunnel: 100.0 ("CCD Chip Vertical End") -> [w42]
        tunnel: 1.0 ("Horizontal Binning") -> [w41]
        frame #0 {
          n8 = global write "GlobalSetGetConfigureCamera.vi" "Hbin"(w41) -> ()
          n9 = global write "GlobalSetGetConfigureCamera.vi" "Vbin"(w44) -> ()
          n10 = global write "GlobalSetGetConfigureCamera.vi" "Vbin"(w45) -> ()
          n11 = Subtract(x=w43, y=w44) -> (x-y=w47:dbl)
          n12 = Subtract(x=w42, y=w40) -> (x-y=w46:dbl)
          n13 = global write "ccdChipPixels.vi" "CCD Chip Vertical end"(w42) -> ()
          n14 = global write "ccdChipPixels.vi" "CCD Chip Vertical Start"(w40) -> ()
          n15 = global write "ccdChipPixels.vi" "CCD Chip horizontal end"(w43) -> ()
          n16 = global write "ccdChipPixels.vi" "CCD Chip horizontal start"(w40) -> ()
          n17 = Increment(x=w47) -> (x+1=w49:dbl)
          n18 = Increment(x=w46) -> (x+1=w48:dbl)
          n19 = Multiply(x=w49, y=w48) -> (x*y=w50:dbl)
          n20 = global write "ccdChipPixels.vi" "CCD Chip Size"(w50) -> ()
        }
      }
      n21 = property on="Aquire Image" class="Bool"("BoolText.Text"="Aquire Image" ("Caption.Text"), "BoolText.TextColor"=u32 0 ("Boolean Text.Colors:FG Color")) -> ()  [unwired: 2 in, 2 out]
      n22 = local write "PI SystemNumber"(1 ("PI SystemNumber")) -> ()
      n23 = property on="Point Measurement" class="Bool"("BoolText.Text"="Point Measurement" ("Caption.Text"), "BoolText.TextColor"=u32 0 ("Boolean Text.Colors:FG Color")) -> ()  [unwired: 2 in, 2 out]
      n24 = call "MTS_ClearWSTree2.vi"("error in"=w31, "Tree Refnum"=w38) -> ("error out"=w20:errorcluster)  [unwired: 8 in, 1 out]
      "Global Stop" <- w39
      "Running" <- w39
      "Buffer Overrun" <- w39
      "Stop Measurement" <- w39
      "Workspace" <- w32
      "Active pt3" <- w32
      "Task" <- T10."No Measurement" ("Do Measurement")
    }
  }
  n25 = local read "PI SystemNumber"() -> (w9:i32)
  n26 = control-ref of="X-Position"() -> (w13:refnum<vi>)
  n27 = control-ref of="Y-Position"() -> (w12:refnum<vi>)
  n28 = control-ref of="Z-Position"() -> (w11:refnum<vi>)
  n29 = call "AndorPhysikInstrumenteInitialisiation.vi"("reference"=w13, "error in (no error)"=w14, "reference 3"=w11, "reference 2"=w12, "Pi"=w9) -> ("error out"=w6:errorcluster, "Device List"=w18:T12)  [unwired: 5 in]
  n30 = while {
    shift-right: [w54] -> _
    shift-left: w6 -> [w55]
    stop <- w52 stop-if-true
    n31 = Wait (ms)(milliseconds to wait=u32 100) -> ()  [unwired: 1 out]
    n32 = local read "Global Stop"() -> (w52:bool)
    n33 = control-ref of="Point"() -> (w51:refnum<vi>)
    n34 = call "RunCameraPreview.vi"("error in (no error)"=w55, "Point 2"=w51) -> ("error out"=w54:errorcluster)  [unwired: 9 in]
  }
  n35 = while {
    tunnel: w6 -> [w72]
    stop <- w58 stop-if-true
    n36 = local read "Global Stop"() -> (w73:bool)
    n37 = local read "Global Stop"() -> (w58:bool)
    n38 = call "Vision Acquisition"("Auto Exposure::Mode"="Auto Exposure::Mode", "Auto Exposure::Value"="Auto Exposure::Value", "Brightness::Mode"="Brightness::Mode", "Brightness::Value"="Brightness::Value", "Gain::Mode"="Gain::Mode", "Stop (F)"=w73, "Gain::Value"="Gain::Value", "error in"=w72, "Gamma::Mode"="Gamma::Mode", "Shutter::Mode"="Shutter::Mode", "Shutter::Value"="Shutter::Value", "Trigger::Trigger Activation"="Trigger::Trigger Activation", "Trigger::Trigger Mode"="Trigger::Trigger Mode", "Trigger::Trigger Parameter"="Trigger::Trigger Parameter", "Trigger Delay::Mode"="Trigger Delay::Mode") -> ("Image Out"=→"Image Out":T5, "Image Number"=→"Image Number":u32, "Frame Rate"=→"acquired FPS":dbl)  [unwired: 8 in, 2 out]
  }
  n39 = while {
    shift-right: [w113] -> _
    shift-left: w6 -> [w115]
    stop <- w114 stop-if-true
    n40 = local read "Global Stop"() -> (w114:bool)
    n41 = control-ref of="WS File Tree"() -> (w88:refnum<vi>)
    n42 = global read "GlobalLaserInterface.vi" "InterfaceLaserInitalised"() -> (w76:refnum<visa-resource-name>)
    n43 = event shown="[10] \"X-Position\", \"Y-Position\", \"Z-Position\": Value Change;  \"Move Stage\": Mouse Up" {
      selector: _ -> [_ _ _ _ _ _ _ _ _ _ _ _ _ _ _ _ _ _ _ _ _ _ _ _ _ _ _ _ _]
      dyn-events: _ -> [_ _ _ _ _ _ _ _ _ _ _ _ _ _ _ _ _ _ _ _ _ _ _ _ _ _ _ _ _]
      timeout: _ -> [_ _ _ _ _ _ _ _ _ _ _ _ _ _ _ _ _ _ _ _ _ _ _ _ _ _ _ _ _]
      tunnel: w115 -> [w116 w118 _ _ w193 _ w236 _ _ _ w279 w332 w335 w371 _ w431 _ w471 w478 w507 _ w517 w526 w537 w539 _ _ _ w546]
      tunnel: [w116 w118 _ _ w194 _ w235 _ _ _ w278 w324 w333 w368 _ w430 _ w470 _ _ _ w515 _ w536 _ _ _ _ w547] -> w113
      tunnel: w88 -> [_ _ _ _ _ _ _ _ _ _ _ _ w337 w372 _ _ _ _ _ _ _ _ _ _ _ _ _ _ _]
      tunnel: "Aquire Image" -> [_ _ _ _ _ _ _ _ _ _ _ _ _ _ _ _ _ _ _ _ _ _ _ _ _ _ _ _ _]
      tunnel: "Save Color Image" -> [_ _ _ _ _ _ _ _ _ _ _ _ _ _ _ _ _ _ _ _ _ _ _ _ _ _ _ _ _]
      tunnel: "Open MSW" -> [_ _ _ _ _ _ _ _ _ _ _ _ _ _ _ _ _ _ _ _ _ _ _ _ _ _ _ _ _]
      tunnel: "Find Mols" -> [_ _ _ _ _ _ _ _ _ _ _ _ _ _ _ _ _ _ _ _ _ _ _ _ _ _ _ _ _]
      tunnel: "Auto Meas" -> [_ _ _ _ _ _ _ _ _ _ _ _ _ _ _ _ _ _ _ _ _ _ _ _ _ _ _ _ _]
      tunnel: "New MSW" -> [_ _ _ _ _ _ _ _ _ _ _ _ _ _ _ _ _ _ _ _ _ _ _ _ _ _ _ _ _]
      tunnel: "Stop Program" -> [_ _ _ _ _ _ _ _ _ _ _ _ _ _ _ _ _ _ _ _ _ _ _ _ _ _ _ _ _]
      tunnel: "Point Measurement" -> [_ _ _ _ _ _ _ _ _ _ _ _ _ _ _ _ _ _ _ _ _ _ _ _ _ _ _ _ _]
      tunnel: "Move Stage" -> [_ _ _ _ _ _ _ _ _ _ _ _ _ _ _ _ _ _ _ _ _ _ _ _ _ _ _ _ _]
      tunnel: w76 -> [_ _ _ _ _ _ _ _ _ _ _ _ _ _ _ _ _ _ _ _ _ _ _ _ _ _ _ _ _]
      tunnel: "Get Position" -> [_ _ _ _ _ _ _ _ _ _ _ _ _ _ _ _ _ _ _ _ _ _ _ _ _ _ _ _ _]
      tunnel: [_ _ _ _ _ _ _ _ _ _ w274 w317 _ _ _ _ _ _ _ _ _ _ _ _ _ _ _ _ _] -> w103
      tunnel: [_ _ _ _ _ _ _ _ _ _ w275 w318 _ _ _ _ _ _ _ _ _ _ _ _ _ _ _ _ _] -> w87
      tunnel: [_ _ _ _ _ _ _ _ _ _ w276 w319 _ _ _ _ _ _ _ _ _ _ _ _ _ _ _ _ _] -> w102
      tunnel: "How long?" -> [_ _ _ _ _ _ _ _ _ _ _ _ _ _ _ _ _ _ _ _ _ _ _ _ _ _ _ _ _]
      tunnel: "Start 3D FCS Abel Scan" -> [_ _ _ _ _ _ _ _ _ _ _ _ _ _ _ _ _ _ _ _ _ _ _ _ _ _ _ _ _]
      tunnel: "Mesaurement Time (Sec) / Step" -> [_ _ _ w152 w198 _ _ _ _ _ _ _ _ _ _ _ _ _ _ _ _ _ _ _ _ _ w544 _ _]
      tunnel: "Y Stepsize" -> [_ _ _ w151 w197 _ _ _ _ _ _ _ _ _ _ _ _ _ _ _ _ _ _ _ _ _ _ _ _]
      tunnel: "X Stepsize" -> [_ _ _ w150 w196 _ _ _ _ _ _ _ _ _ _ _ _ _ _ _ _ _ _ _ _ _ _ _ _]
      tunnel: "Z Stepsize" -> [_ _ _ w149 w195 _ _ _ _ _ _ _ _ _ _ _ _ _ _ _ _ _ _ _ _ _ _ _ _]
      tunnel: "FCS Point Measurement" -> [_ _ _ _ _ _ _ _ _ _ _ _ _ _ _ _ _ _ _ _ _ _ _ _ _ _ _ _ _]
      tunnel: "Z End" -> [_ _ _ w148 w207 _ _ _ _ _ _ _ _ _ _ _ _ _ _ _ _ _ _ _ _ _ _ _ _]
      tunnel: "X End" -> [_ _ _ w147 w201 _ _ _ _ _ _ _ _ _ _ _ _ _ _ _ _ _ _ _ _ _ _ _ _]
      tunnel: "Y End" -> [_ _ _ w146 w204 _ _ _ _ _ _ _ _ _ _ _ _ _ _ _ _ _ _ _ _ _ _ _ _]
      tunnel: "Z Start" -> [_ _ _ w145 w187 _ _ _ _ _ _ _ _ _ _ _ _ _ _ _ _ _ _ _ _ _ _ _ _]
      tunnel: "X Start" -> [_ _ _ w144 w189 _ _ _ _ _ _ _ _ _ _ _ _ _ _ _ _ _ _ _ _ _ _ _ _]
      tunnel: "Y Start" -> [_ _ _ w143 w188 _ _ _ _ _ _ _ _ _ _ _ _ _ _ _ _ _ _ _ _ _ _ _ _]
      tunnel: w88 -> [_ _ _ _ _ _ _ _ _ _ _ _ _ _ _ _ _ _ _ _ _ _ _ _ _ _ _ _ _]
      tunnel: "SET CCD" -> [_ _ _ _ _ _ _ _ _ _ _ _ _ _ _ _ _ _ _ _ _ _ _ _ _ _ _ _ _]
      tunnel: "OPEN SHUTER" -> [_ _ _ _ _ _ _ _ _ _ _ _ _ _ _ _ _ _ _ _ _ w516 _ _ _ _ _ _ _]
      tunnel: "Close" -> [_ _ _ _ _ _ _ _ _ _ _ _ _ _ _ _ _ _ _ _ _ _ w525 _ _ _ _ _ _]
      tunnel: "Stop" -> [_ _ _ _ _ _ _ _ _ _ _ _ _ _ _ _ _ _ _ _ _ _ _ _ _ _ _ _ _]
      tunnel: "Start" -> [_ _ _ _ _ _ _ _ _ _ _ _ _ _ _ _ _ _ _ _ _ _ _ _ _ _ _ _ _]
      tunnel: "Gain" -> [_ _ _ _ _ _ _ _ _ _ _ _ _ _ _ _ _ _ _ _ _ _ _ _ _ _ _ _ _]
      tunnel: "Cam (Defocused)" -> [_ _ _ _ _ _ _ _ _ _ _ _ _ _ _ _ _ _ _ _ w514 _ _ _ _ _ _ _ _]
      tunnel: "Set Temperature" -> [_ _ _ _ _ _ _ _ _ _ _ _ _ _ _ _ _ _ _ _ _ _ _ _ _ _ _ _ _]
      tunnel: "SCANNER EMERGENCY" -> [_ _ _ _ _ _ _ _ _ _ _ _ _ _ _ _ _ _ _ _ _ _ _ _ _ _ _ _ _]
      tunnel: "Get Temperature" -> [_ _ _ _ _ _ _ _ _ _ _ _ _ _ _ _ _ _ _ _ _ _ _ _ _ _ _ _ _]
      event Timeout {
        n44 = event-data() -> ()  [unwired: 1 in, 2 out]
      }
      event "Stop Program": Mouse Up {
        n45 = event-data() -> ()  [unwired: 1 in, 7 out]
        n46 = local write "Global Stop"(TRUE ("Global Stop")) -> ()
      }
      event "Aquire Image": Mouse Up {
        n47 = event-data() -> ()  [unwired: 1 in, 7 out]
        n48 = local read "Workspace"() -> (w122:path)
        n49 = local read "Running"() -> (w125:bool)
        n50 = Not(x=w125) -> (.not. x?=w124:bool)
        n51 = Not Equal?(x=w122, y=path "") -> (x != y?=w120:bool)
        n52 = local read "Task"() -> (w119:T10)
        n53 = case shown="True" w120 {
          tunnel: w124 -> [_ w129]
          tunnel: T13."Aquire Image" ("Do Measurement") -> [_ w128]
          tunnel: w119 -> [_ w127]
          frame False {
            # "No Workspace Open"
            n54 = One Button Dialog(message="No Workspace Opened") -> ()  [unwired: 1 in, 1 out]
          }
          frame True {
            # "Aquire Image if not Running"
            n55 = case shown="True" w129 {
              tunnel: w128 -> [w132 w135]
              tunnel: w127 -> [w130 _]
              frame False {
                n56 = Equal?(x=w130, y=w132) -> (x = y?=w131:bool)
                n57 = case shown="False" w131 {
                  frame False {
                  }
                  frame True {
                    n58 = local write "Stop Measurement"(TRUE ("Stop Measurement")) -> ()
                  }
                }
              }
              frame True {
                n59 = local write "Task"(w135) -> ()
                n60 = local write "Running"(TRUE ("Measurement Running")) -> ()
                n61 = property on="Aquire Image" class="Bool"("BoolText.Text"="Stop Aquire" ("Caption.Text"), "BoolText.TextColor"=u32 16711680 ("Boolean Text.Colors:FG Color")) -> ()  [unwired: 2 in, 2 out]
              }
            }
          }
        }
      }
      event "How long?": Value Change {
        n62 = event-data() -> ()  [unwired: 1 in, 5 out]
        n63 = Build Array(w152, w151, w150, w149, w148, w147, w146, w145, w144, w143) -> (w142:dbl[])
        n64 = for {
          tunnel: w142 -> [w180] mode=indexing
          tunnel: [w179] -> w141 mode=indexing
          n65 = Not Equal To 0?(x=w180) -> (x != 0?=w179:bool)
        }
        n66 = Boolean Array To Number(Boolean array=w141) -> (number=w140:u32)
        n67 = Not Equal To 0?(x=w140) -> (x != 0?=w139:bool)
        n68 = case shown="True" w139 {
          tunnel: [0.0 w165] -> w138
          tunnel: w152 -> [_ w164]
          tunnel: w151 -> [_ w163]
          tunnel: w150 -> [_ w162]
          tunnel: w149 -> [_ w161]
          tunnel: w148 -> [_ w160]
          tunnel: w147 -> [_ w159]
          tunnel: w146 -> [_ w158]
          tunnel: w145 -> [_ w157]
          tunnel: w144 -> [_ w156]
          tunnel: w143 -> [_ w155]
          frame False {
            n69 = One Button Dialog(message="Supply valid information for the scanner x-z and stepsize and apply a measurement time ") -> ()  [unwired: 1 in, 1 out]
          }
          frame True {
            w166 = 60.0 ("y")
            # "to hours"
            # "to minutes"
            n70 = Subtract(x=w160, y=w157) -> (x-y=w173:dbl)
            n71 = Subtract(x=w159, y=w156) -> (x-y=w178:dbl)
            n72 = Subtract(x=w158, y=w155) -> (x-y=w175:dbl)
            n73 = Divide(x=w173, y=w161) -> (x/y=w174:dbl)
            n74 = Divide(x=w178, y=w162) -> (x/y=w177:dbl)
            n75 = Divide(x=w175, y=w163) -> (x/y=w176:dbl)
            n76 = Multiply(x=w164, y=w174) -> (x*y=w170:dbl)
            n77 = Multiply(x=w164, y=w177) -> (x*y=w172:dbl)
            n78 = Multiply(x=w164, y=w176) -> (x*y=w171:dbl)
            n79 = Add(x=w172, y=w171) -> (x+y=w169:dbl)
            n80 = Add(x=w170, y=w169) -> (x+y=w168:dbl)
            n81 = Divide(x=w168, y=w166) -> (x/y=w167:dbl)
            n82 = Divide(x=w167, y=w166) -> (x/y=w165:dbl)
          }
        }
        "Estimated Time (h)" <- w138
      }
      event "Start 3D FCS Abel Scan": Value Change {
        w190 = 200
        n83 = event-data() -> ()  [unwired: 1 in, 5 out]
        n84 = local write "Z Stepsize"(w195) -> ()
        n85 = local write "X-Position"(w189) -> ()
        n86 = local write "Y-Position"(w188) -> ()
        n87 = local write "Y Stepsize"(w197) -> ()
        n88 = property on="Measurement Time" class="DigNum (strict)"("Value"=w198) -> ()  [unwired: 2 in, 2 out]
        n89 = local write "Z-Position"(w187) -> ()
        n90 = local write "X Stepsize"(w196) -> ()
        n91 = case shown="No Error" w193 {
          selector: w193 -> [w208 w210]
          tunnel: [w208 w210] -> w182
          frame No Error {
            n92 = global write "StopGetPic.vi" "Stop"(TRUE ("Stop")) -> ()
          }
          frame Error {
          }
        }
        n93 = Subtract(x=w201, y=w189) -> (x-y=w200:dbl)
        n94 = Subtract(x=w207, y=w187) -> (x-y=w205:dbl)
        n95 = Subtract(x=w204, y=w188) -> (x-y=w203:dbl)
        n96 = Divide(x=w200, y=w196) -> (x/y=→"X Steps":dbl)
        n97 = Divide(x=w205, y=w195) -> (x/y=→"Z Steps":dbl)
        n98 = Divide(x=w203, y=w197) -> (x/y=→"Y Steps":dbl)
        n99 = local read "PI SystemNumber"() -> (w192:i32)
        n100 = Subtract(x=w190, y=w187) -> (x-y=w184:dbl)
        n101 = Subtract(x=w190, y=w188) -> (x-y=w185:dbl)
        n102 = Subtract(x=w190, y=w189) -> (x-y=w186:dbl)
        n103 = Build Array(w186, w185, w184) -> (w183:dbl[])
        n104 = global read "GlobalConAxisPI.vi" "Conn. Axes"() -> (w191:string[])
        n105 = call "MOV.vi"("System no."=w192, "Axes to move"=w191, "Position values"=w183, "error in"=w182) -> ("error out"=w181:errorcluster)  [unwired: 15 in]
        n106 = case shown="No Error" w181 {
          selector: w181 -> [w211 w213]
          tunnel: [w211 w213] -> w194
          frame No Error {
            "3dAbelFcs" <- TRUE
          }
          frame Error {
          }
        }
      }
      event "Auto Meas": Mouse Up {
        n107 = event-data() -> ()  [unwired: 1 in, 7 out]
        n108 = local read "Workspace"() -> (w221:path)
        n109 = local read "Running"() -> (w224:bool)
        n110 = local read "Last Image File No"() -> (w218:i32)
        n111 = Not(x=w224) -> (.not. x?=w223:bool)
        n112 = Not Equal?(x=w221, y=path "") -> (x != y?=w216:bool)
        n113 = Not Equal?(x=w218, y=-1) -> (x != y?=w215:bool)
        n114 = And(x=w216, y=w215) -> (x .and. y?=w214:bool)
        n115 = local read "Task"() -> (w222:T10)
        n116 = case shown="False" w214 {
          tunnel: w223 -> [_ w228]
          tunnel: T14."Auto Measurement Control" ("Do Measurement") -> [_ w227]
          tunnel: w222 -> [_ w226]
          frame False {
            # "No Workspace Open"
            n117 = One Button Dialog(message="No Workspace Opened or No Image Acquired") -> ()  [unwired: 1 in, 1 out]
          }
          frame True {
            # "Start Auto Measurement"
            n118 = case shown="True" w228 {
              tunnel: w227 -> [_ w232]
              tunnel: w226 -> [_ _]
              frame False {
                n119 = case shown="True" FALSE {
                  frame False {
                  }
                  frame True {
                    n120 = local write "Stop Measurement"(TRUE ("Stop Measurement")) -> ()
                  }
                }
              }
              frame True {
                n121 = local write "Task"(w232) -> ()
                n122 = local write "Running"(TRUE ("Measurement Running")) -> ()
                n123 = local write "NxtAutMesPoint"(-1 ("NxtAutMesPoint")) -> ()
              }
            }
          }
        }
      }
      event "Get Temperature": Value Change {
        n124 = event-data() -> ()  [unwired: 1 in, 5 out]
        n125 = call "GetTemperature.vi"("error in (no error)"=w236) -> ("error out"=w237:errorcluster, "temperature"=w240:i32)  [unwired: 3 in, 2 out]
        n126 = call "Build Text"("Cam"=w240, "error in (no error)"=w237) -> ("Result"=w239:string, "error out"=w238:errorcluster)  [unwired: 12 in]
        n127 = call "Display Message to User"("error in (no error)"=w238, "Enable"=TRUE, "Message"=w239) -> ("error out"=w235:errorcluster)  [unwired: 7 in, 1 out]
      }
      event "Save Color Image": Mouse Up {
        n128 = event-data() -> ()  [unwired: 1 in, 7 out]
        n129 = local read "Active pt3"() -> (w243:path)
        n130 = Not Equal?(x=w243, y=path "") -> (x != y?=w241:bool)
        n131 = case shown="True" w241 {
          tunnel: T15."Save Color Image" ("Do Measurement") -> [_ w247]
          frame False {
            # "No Workspace Open"
            n132 = One Button Dialog(message="No pt3 File opened") -> ()  [unwired: 1 in, 1 out]
          }
          frame True {
            # "Aquire Image if not Running"
            n133 = local write "Task"(w247) -> ()
            n134 = local write "Running"(TRUE ("Measurement Running")) -> ()
          }
        }
      }
      event "Find Mols": Mouse Up {
        n135 = event-data() -> ()  [unwired: 1 in, 7 out]
        n136 = local read "Active pt3"() -> (w250:path)
        n137 = Not Equal?(x=w250, y=path "") -> (x != y?=w248:bool)
        n138 = case shown="True" w248 {
          tunnel: T15."Find Single Mol." ("Do Measurement") -> [_ w254]
          frame False {
            # "No Workspace Open"
            n139 = One Button Dialog(message="No pt3 File opened") -> ()  [unwired: 1 in, 1 out]
          }
          frame True {
            # "Aquire Image if not Running"
            n140 = local write "Task"(w254) -> ()
            n141 = local write "Running"(TRUE ("Measurement Running")) -> ()
          }
        }
      }
      event "Point Measurement": Mouse Up {
        n142 = event-data() -> ()  [unwired: 1 in, 7 out]
        n143 = local read "Workspace"() -> (w257:path)
        n144 = local read "Running"() -> (w261:bool)
        n145 = Not(x=w261) -> (.not. x?=w260:bool)
        n146 = Not Equal?(x=w257, y=path "") -> (x != y?=w255:bool)
        n147 = local read "Task"() -> (w258:T10)
        n148 = case shown="True" w255 {
          tunnel: w260 -> [_ w265]
          tunnel: T13."Point Measurement" ("Do Measurement") -> [_ w264]
          tunnel: w258 -> [_ w263]
          frame False {
            # "No Workspace Open"
            n149 = One Button Dialog(message="No Workspace Opened") -> ()  [unwired: 1 in, 1 out]
          }
          frame True {
            # "Aquire Image if not Running"
            n150 = case shown="False" w265 {
              tunnel: w264 -> [w267 w271]
              tunnel: w263 -> [w268 _]
              frame False {
                n151 = Equal?(x=w268, y=w267) -> (x = y?=w266:bool)
                n152 = case shown="False" w266 {
                  frame False {
                  }
                  frame True {
                    n153 = local write "Stop Measurement"(TRUE ("Stop Measurement")) -> ()
                  }
                }
              }
              frame True {
                n154 = local write "Task"(w271) -> ()
                n155 = local write "Running"(TRUE ("Measurement Running")) -> ()
                n156 = property on="Point Measurement" class="Bool"("BoolText.Text"="Stop Aquire" ("Caption.Text"), "BoolText.TextColor"=u32 16711680 ("Boolean Text.Colors:FG Color")) -> ()  [unwired: 2 in, 2 out]
              }
            }
          }
        }
      }
      event "X-Position", "Y-Position", "Z-Position": Value Change; "Move Stage": Mouse Up {
        n157 = event-data() -> ()  [unwired: 1 in, 3 out]
        n158 = local read "Workspace"() -> (w282:path)
        n159 = local read "Running"() -> (w284:bool)
        n160 = local read "PI SystemNumber"() -> (w277:i32)
        n161 = Not(x=w284) -> (.not. x?=w283:bool)
        n162 = Not Equal?(x=w282, y=path "") -> (x != y?=w280:bool)
        n163 = case shown="True" w280 {
          tunnel: w283 -> [_ w292]
          tunnel: w279 -> [_ w291]
          tunnel: [_ w290] -> w278
          tunnel: w277 -> [_ w289]
          tunnel: [_ w288] -> w274
          tunnel: [_ w287] -> w275
          tunnel: [_ w286] -> w276
          frame False {
            # "No Workspace Open"
            n164 = One Button Dialog(message="No Workspace Opened") -> ()  [unwired: 1 in, 1 out]
          }
          frame True {
            # "Move Stage if not Running"
            n165 = case shown="True" w292 {
              tunnel: w291 -> [_ w316]
              tunnel: [_ w306] -> w290
              tunnel: w289 -> [_ w314]
              tunnel: [_ w293] -> w288
              tunnel: [_ w294] -> w287
              tunnel: [_ w295] -> w286
              frame False {
              }
              frame True {
                w298 = 200
                n166 = local read "X-Position"() -> (w301:dbl)
                n167 = local read "Y-Position"() -> (w300:dbl)
                n168 = local read "Z-Position"() -> (w305:dbl)
                n169 = Subtract(x=w298, y=w301) -> (x-y=w302:dbl)
                n170 = Subtract(x=w298, y=w300) -> (x-y=w303:dbl)
                n171 = Subtract(x=w298, y=w305) -> (x-y=w304:dbl)
                n172 = Build Array(w302, w303, w304) -> (w315:dbl[])
                n173 = global read "GlobalConAxisPI.vi" "Conn. Axes"() -> (w313:string[])
                n174 = call "MOV.vi"("System no."=w314, "Axes to move"=w313, "Position values"=w315, "error in"=w316) -> ("error out"=w311:errorcluster)  [unwired: 15 in]
                n175 = call "POS?.vi"("System no."=w314, "Axes to query"=w313, "All axes?"=TRUE, "error in"=w311) -> ("Position"=w310:dbl[], "error out"=w306:errorcluster)  [unwired: 14 in]
                n176 = Index Array(array=w310, index #1=0 ("index"), index #2=1 ("index"), index #3=2 ("index")) -> (element #1=w299:dbl, element #2=w296:dbl, element #3=w297:dbl)
                n177 = Subtract(x=w298, y=w299) -> (x-y=w295:dbl)
                n178 = Subtract(x=w298, y=w296) -> (x-y=w294:dbl)
                n179 = Subtract(x=w298, y=w297) -> (x-y=w293:dbl)
              }
            }
          }
        }
        n180 = property on="y-position" class="DigNum (strict)"("Value"=w275) -> ()  [unwired: 2 in, 2 out]
        n181 = property on="z-position" class="DigNum (strict)"("Value"=w274) -> ()  [unwired: 2 in, 2 out]
        n182 = property on="x-position" class="DigNum (strict)"("Value"=w276) -> ()  [unwired: 2 in, 2 out]
      }
      event "Get Position": Value Change {
        w323 = 200
        n183 = event-data() -> ()  [unwired: 1 in, 5 out]
        n184 = local read "PI SystemNumber"() -> (w331:i32)
        n185 = global read "GlobalConAxisPI.vi" "Conn. Axes"() -> (w330:string[])
        n186 = call "POS?.vi"("System no."=w331, "Axes to query"=w330, "All axes?"=TRUE, "error in"=w332) -> ("Position"=w328:dbl[], "error out"=w324:errorcluster)  [unwired: 14 in]
        n187 = Index Array(array=w328, index #1=0 ("index"), index #2=1 ("index"), index #3=2 ("index")) -> (element #1=w320:dbl, element #2=w321:dbl, element #3=w322:dbl)
        n188 = Subtract(x=w323, y=w320) -> (x-y=w319:dbl)
        n189 = Subtract(x=w323, y=w321) -> (x-y=w318:dbl)
        n190 = Subtract(x=w323, y=w322) -> (x-y=w317:dbl)
        n191 = property on="y-position" class="DigNum (strict)"("Value"=w318) -> ()  [unwired: 2 in, 2 out]
        n192 = property on="x-position" class="DigNum (strict)"("Value"=w319) -> ()  [unwired: 2 in, 2 out]
        n193 = property on="z-position" class="DigNum (strict)"("Value"=w317) -> ()  [unwired: 2 in, 2 out]
      }
      event "New MSW": Mouse Up {
        # "Default Name"
        n194 = event-data() -> ()  [unwired: 1 in, 7 out]
        n195 = flat-sequence {
          tunnel: [w353] -> w336
          tunnel: w335 -> [w353]
          frame #0 {
            n196 = local write "Running"(TRUE ("MeasRunig")) -> ()
          }
        }
        n197 = Get Date/Time In Seconds() -> (seconds since 1Jan1904=w350:timestamp)
        n198 = Format Date/Time String(time format string (%c)="%Y-%m-%d", seconds (now)=w350) -> (date/time string=w348:string)  [unwired: 1 out]
        n199 = Concatenate Strings(w348, ".msw" ("string")) -> (w346:string)
        n200 = call "File Dialog"("start path"=path "D:/", "prompt"="Create New Workspace", "button label"="Create", "default name"=w346, "error in"=w336, "pattern (all files)"="*.msw", "pattern label"="MT Scan Workspace") -> ("selected path"=w340:path, "cancelled"=w341:bool, "error out"=w339:errorcluster)  [unwired: 5 in, 1 out]
        n201 = case shown="False" w341 {
          tunnel: w340 -> [w359 _]
          tunnel: w339 -> [w365 w367]
          tunnel: [w357 w366] -> w334
          tunnel: w337 -> [w355 _]
          frame False {
            # "Create Empty Workspace"
            n202 = local write "Workspace"(w359) -> ()
            n203 = call "MTS_CreateWriteMSW.vi"("Rewrite"=TRUE, "error in (no error)"=w365, "Workspace Path"=w359) -> ("error out"=w358:errorcluster, "Created"=w362:string, "Comment (dup)"=w361:string, "Files in Workspace (dup)"=w360:T19)  [unwired: 5 in]
            n204 = call "MTS_Workspace.vi"("Workspace"=w359, "Operation"=T16."Set Workspace", "Created in"=w362, "New Comment"=w361, "Files in Workspace in"=w360) -> ("Files in Workspace"=w356:T20)  [unwired: 3 in, 3 out]
            n205 = call "MTS_BuildWSTree.vi"("error in"=w358, "Files in Workspace"=w356, "Tree Refnum"=w355) -> ("error out"=w357:errorcluster)  [unwired: 6 in, 2 out]
          }
          frame True {
            n206 = call <vilib>:"Clear Errors.vi"("error in (no error)"=w367) -> ("error out"=w366:errorcluster)  [unwired: 6 in]
          }
        }
        n207 = flat-sequence {
          tunnel: w334 -> [w351]
          tunnel: [w351] -> w333
          frame #0 {
            n208 = local write "Running"(FALSE ("MeasRunig")) -> ()
          }
        }
      }
      event "Open MSW": Mouse Up {
        n209 = event-data() -> ()  [unwired: 1 in, 7 out]
        n210 = flat-sequence {
          tunnel: w371 -> [w383]
          tunnel: [w383] -> w370
          frame #0 {
            n211 = local write "Running"(TRUE ("MeasRunig")) -> ()
          }
        }
        n212 = call "File Dialog2"("start path"=path "D:/", "prompt"="Create New Workspace", "button label"="Open", "error in"=w370, "pattern (all files)"="*.msw", "pattern label"="MT Scan Workspace") -> ("selected path"=w375:path, "cancelled"=w376:bool, "error out"=w374:errorcluster)  [unwired: 6 in, 1 out]
        n213 = case shown="False" w376 {
          tunnel: w375 -> [w391 _]
          tunnel: w374 -> [w396 w398]
          tunnel: [w389 w397] -> w369
          tunnel: w372 -> [w388 _]
          frame False {
            # "Open Workspace"
            n214 = local write "Workspace"(w391) -> ()
            n215 = call "MTS_ReadMSW.vi"("error in (no error)"=w396, "Workspace Path"=w391) -> ("error out"=w390:errorcluster, "Created"=w394:string, "Comment"=w393:string, "Files in Workspace"=w392:T21)  [unwired: 6 in]
            n216 = call "MTS_Workspace.vi"("Workspace"=w391, "Operation"=T16."Set Workspace", "Created in"=w394, "New Comment"=w393, "Files in Workspace in"=w392) -> ("Files in Workspace"=w387:T20)  [unwired: 3 in, 3 out]
            n217 = Array To Cluster(array=w387) -> (cluster=w386:T22)
            n218 = Unbundle By Name(w386) -> ()  [unwired: 1 out]
            n219 = call "MTS_BuildWSTree.vi"("error in"=w390, "Files in Workspace"=w387, "Tree Refnum"=w388) -> ("error out"=w389:errorcluster, "numberOfFilesInWorkspace"=w385:i32)  [unwired: 6 in, 1 out]
            n220 = local write "Last Image File No"(w385) -> ()
          }
          frame True {
            n221 = call <vilib>:"Clear Errors.vi"("error in (no error)"=w398) -> ("error out"=w397:errorcluster)  [unwired: 6 in]
          }
        }
        n222 = flat-sequence {
          tunnel: w369 -> [w381]
          tunnel: [w381] -> w368
          frame #0 {
            n223 = local write "Running"(FALSE ("MeasRunig")) -> ()
          }
        }
      }
      event "Image": Mouse Up {
        w401 = 100.0 ("y")
        n224 = event-data() -> ("Coords"=w413:T23, "PlatMods"=w414:T24)  [unwired: 1 in, 5 out]
        n225 = invoke on="Image" class="IntGraph (strict)" method="Map Coords To XY"("Coords"=w413) -> ("Map Coords To XY"=w410:bool, "XY"=w408:cluster{"X":dbl, "Y":dbl})  [unwired: 6 in, 5 out]
        n226 = Unbundle By Name(w414) -> ("Ctrl"=w411:bool)
        n227 = And(x=w410, y=w411) -> (x .and. y?=w412:bool)
        n228 = Unbundle(w408) -> ("X"=w407:dbl, "Y"=w404:dbl)
        n229 = Multiply(x=w407, y=w401) -> (x*y=w406:dbl)
        n230 = Multiply(x=w404, y=w401) -> (x*y=w403:dbl)
        n231 = Round To Nearest(number=w406) -> (nearest integer value=w405:dbl)
        n232 = Round To Nearest(number=w403) -> (nearest integer value=w402:dbl)
        n233 = Divide(x=w405, y=w401) -> (x/y=w400:dbl)
        n234 = Divide(x=w402, y=w401) -> (x/y=w399:dbl)
        n235 = local read "Axis"() -> (w409:enum32{"x-y", "x-z", "y-x", "y-z", "z-x", "z-y"})
        n236 = case shown="True" w412 {
          tunnel: w409 -> [_ w417]
          tunnel: w400 -> [_ w416]
          tunnel: w399 -> [_ w415]
          frame False {
          }
          frame True {
            n237 = case shown="\"x-y\", Default" w417 {
              tunnel: w416 -> [w419 w421 w423]
              tunnel: w415 -> [w418 w420 w422]
              frame "x-y", Default {
                n238 = local write "X-Position"(w419) -> ()
                n239 = local write "Y-Position"(w418) -> ()
              }
              frame "x-z" {
                n240 = local write "X-Position"(w421) -> ()
                n241 = local write "Z-Position"(w420) -> ()
              }
              frame "y-z" {
                n242 = local write "Y-Position"(w423) -> ()
                n243 = local write "Z-Position"(w422) -> ()
              }
            }
          }
        }
      }
      event "WS File Tree": Value Change {
        n244 = event-data() -> ("NewVal"=w432:string)  [unwired: 1 in, 4 out]
        n245 = control-ref of="Workspace"() -> (w429:refnum<vi>)
        n246 = control-ref of="Histogram"() -> (w427:refnum<vi>)
        n247 = control-ref of="Trace"() -> (w426:refnum<vi>)
        n248 = control-ref of="Image"() -> (w425:refnum<vi>)
        n249 = control-ref of="Image"() -> (w424:refnum<vi>)
        n250 = control-ref of="Active pt3"() -> (w428:refnum<vi>)
        n251 = call "CreateNewWSfile.vi"("reference 5"=w424, "NewVal"=w432, "Image"=w425, "reference in"=w428, "error in (no error)"=w431, "reference 4"=w426, "reference 3"=w427, "Path in"=w429) -> ("error out"=w430:errorcluster)  [unwired: 3 in]
      }
      event "Resolution", "Picture size", "Pixel time", "Picture size 2", "Axis", "Laser  Profile": Value Change {
        n252 = event-data() -> ()  [unwired: 1 in, 5 out]
        n253 = local read "Axis"() -> (w453:enum32{"x-y", "x-z", "y-x", "y-z", "z-x", "z-y"})
        n254 = local read "Picture size"() -> (w455:dbl)
        n255 = local read "X-Position"() -> (w450:dbl)
        n256 = local read "Y-Position"() -> (w449:dbl)
        n257 = local read "Z-Position"() -> (w448:dbl)
        n258 = local read "Resolution"() -> (w447:dbl)
        n259 = local read "Pixel time"() -> (w456:dbl)
        n260 = local write "Axis"(w453) -> ()
        n261 = local read "Picture size 2"() -> (w454:dbl)
        n262 = local read "Laser  Profile"() -> (w437:string)
        n263 = local write "Pixel time"(w456) -> ()
        n264 = call "PI_CheckScan.vi"("Picture size"=w455, "Picture size 2"=w454, "Axis"=w453, "x-Position"=w450, "y-Position"=w449, "z-Position"=w448) -> ("Picture size out"=w451:dbl, "Picture size out 2"=w452:dbl)  [unwired: 8 in, 4 out]
        n265 = String To Byte Array(string=w437) -> (unsigned byte array=w435:u8[])
        n266 = local write "Picture size"(w451) -> ()
        n267 = local write "Picture size 2"(w452) -> ()
        n268 = Divide(x=w451, y=w447) -> (x/y=w459:dbl)
        n269 = Divide(x=w452, y=w447) -> (x/y=w460:dbl)
        n270 = Array Size(array=w435) -> (size(s)=w434:i32)
        n271 = Subtract(x=w435, y=48) -> (x-y=w441:i32[])
        n272 = Round Toward +Infinity(x=w459) -> (ceil(x): smallest int >= x=→"x":dbl)
        n273 = Round Toward +Infinity(x=w460) -> (ceil(x): smallest int >= x=→"y":dbl)
        n274 = Initialize Array(4, w434) -> (w445:i32[])
        n275 = Initialize Array(1, w434) -> (w443:i32[])
        n276 = In Range and Coerce(upper limit=w445, x=w441, lower limit=w443) -> (coerced(x)=w438:i32[])  [unwired: 1 out]
        n277 = Add(x=w438, y=48) -> (x+y=w440:i32[])
        n278 = Byte Array To String(unsigned byte array=w440) -> (string=w436:string)
        n279 = while {
          shift-right: [w465] -> w433
          shift-left: w436 -> [w469]
          i -> [w461]
          stop <- w464 stop-if-true
          n280 = Increment(x=w461) -> (x+1=w462:i32)
          n281 = String Subset(string=w469, offset (0)=w461, length (rest)=1) -> (substring=w467:string)
          n282 = Search and Replace String(replace all?=TRUE, input string=w469, search string=w467, offset=w462) -> (result string=w465:string)  [unwired: 4 in, 3 out]
          n283 = String Length(string=w465) -> (length=w463:i32)
          n284 = Less?(x=w463, y=w461) -> (x < y?=w464:bool)
        }
        n285 = local write "Laser  Profile"(w433) -> ()
      }
      event "SCANNER EMERGENCY": Value Change {
        n286 = event-data() -> ()  [unwired: 1 in, 5 out]
        n287 = local read "PI SystemNumber"() -> (w472:i32)
        n288 = call "PI Write GPIB.vi"("System no."=w472, "String to send"="0RT", "error in"=w471) -> ("error out"=w474:errorcluster)  [unwired: 16 in]
        n289 = flat-sequence {
          tunnel: [w475] -> w470
          tunnel: w474 -> [w475]
          frame #0 {
            n290 = One Button Dialog(message="Emergency scanner stop appeared!!!\nCheck scanner settings before continue!!!") -> ()  [unwired: 2 out]
          }
        }
      }
      event "SET CCD": Value Change {
        n291 = event-data() -> ()  [unwired: 1 in, 6 out]
        n292 = call "Camera CCD Chip settings"("error in (no error)"=w478) -> ("Horizontal Binning"=w479:dbl, "Vertical Binning"=w484:dbl, "CCD Chip Horizontal Start"=w483:dbl, "CCD Chip Horizontal End"=w481:dbl, "CCD Chip Vertical Start"=w482:dbl, "CCD Chip Vertical End"=w480:dbl, "OK"=w485:bool, "error out"=w477:errorcluster)  [unwired: 11 in]
        n293 = case shown="True" w485 {
          tunnel: w484 -> [_ w493]
          tunnel: w483 -> [_ w492]
          tunnel: w482 -> [_ w491]
          tunnel: w481 -> [_ w490]
          tunnel: w480 -> [_ w489]
          tunnel: w479 -> [_ w488]
          tunnel: [_ w487] -> _
          tunnel: w477 -> [_ w486]
          frame False {
          }
          frame True {
            n294 = flat-sequence {
              tunnel: w493 -> [w500]
              tunnel: w492 -> [w494]
              tunnel: w491 -> [w499]
              tunnel: w490 -> [w498]
              tunnel: w489 -> [w497]
              tunnel: w488 -> [w496]
              tunnel: [w495] -> w487
              tunnel: w486 -> [w495]
              frame #0 {
                n295 = global write "GlobalSetGetConfigureCamera.vi" "Vbin"(w500) -> ()
                n296 = global write "GlobalSetGetConfigureCamera.vi" "Hbin"(w496) -> ()
                n297 = global write "ccdChipPixels.vi" "CCD Chip Vertical Start"(w499) -> ()
                n298 = global write "ccdChipPixels.vi" "CCD Chip horizontal end"(w498) -> ()
                n299 = global write "ccdChipPixels.vi" "CCD Chip Vertical end"(w497) -> ()
                n300 = global write "ccdChipPixels.vi" "CCD Chip horizontal start"(w494) -> ()
                n301 = Subtract(x=w498, y=w494) -> (x-y=w502:dbl)
                n302 = Subtract(x=w497, y=w499) -> (x-y=w501:dbl)
                n303 = Increment(x=w502) -> (x+1=w504:dbl)
                n304 = Increment(x=w501) -> (x+1=w503:dbl)
                n305 = Multiply(x=w504, y=w503) -> (x*y=w505:dbl)
                n306 = global write "ccdChipPixels.vi" "CCD Chip Size"(w505) -> ()
              }
            }
          }
        }
      }
      event "Set Temperature": Value Change {
        n307 = event-data() -> ()  [unwired: 1 in, 6 out]
        n308 = call "camera cooling"("error in (no error)"=w507) -> ("Temperature"=w508:dbl, "OK"=w509:bool, "error out"=w506:errorcluster)  [unwired: 16 in]
        n309 = case shown="True" w509 {
          tunnel: w508 -> [_ w513]
          tunnel: w506 -> [w510 w512]
          tunnel: [w510 w511] -> _
          frame False {
          }
          frame True {
            n310 = call "CheckTemperature.vi"("error in (no error)"=w512, "temperature in"=w513) -> ("error out"=w511:errorcluster)  [unwired: 9 in]
          }
        }
      }
      event "Cam (Defocused)": Value Change {
        n311 = event-data() -> ()  [unwired: 1 in, 6 out]
        n312 = global write "CamDef.vi" "CamDef"(w514) -> ()
      }
      event "OPEN SHUTER": Value Change {
        n313 = event-data() -> ()  [unwired: 1 in, 6 out]
        n314 = case shown="False" w516 {
          tunnel: [Shutter_mode_typedef."Close" ("mode") Shutter_mode_typedef."Open" ("mode")] -> w520
          tunnel: w517 -> [w522 w523]
          tunnel: [w522 w523] -> w519
          frame False {
          }
          frame True {
          }
        }
        n315 = call "SetShutter.vi"("type"=Shutter_type_typedef."TTL Low", "mode"=w520, "error in (no error)"=w519) -> ("error out"=w515:errorcluster)  [unwired: 11 in, 1 out]
      }
      event "Close": Value Change {
        n316 = event-data() -> ()  [unwired: 1 in, 6 out]
        n317 = case shown="True" w525 {
          tunnel: [Shutter_mode_typedef."Open" ("mode") Shutter_mode_typedef."Open" ("mode")] -> w529
          tunnel: w526 -> [w531 w532]
          tunnel: [w531 w532] -> w528
          frame False {
          }
          frame True {
          }
        }
        n318 = call "SetShutter.vi"("type"=Shutter_type_typedef."TTL Low", "mode"=w529, "error in (no error)"=w528) -> ()  [unwired: 11 in, 2 out]
      }
      event "Exposure": Value Change {
        n319 = event-data() -> ()  [unwired: 1 in, 6 out]
        n320 = call "Camera kinetic settings"("error in (no error)"=w537) -> ("Exposure time"=w534:dbl, "OK"=w535:bool, "error out"=w536:errorcluster)  [unwired: 16 in]
        n321 = case shown="True" w535 {
          tunnel: w534 -> [_ w538]
          frame False {
          }
          frame True {
            n322 = global write "GlobalSetGetConfigureCamera.vi" "Exposure"(w538) -> ()
          }
        }
      }
      event "Gain": Value Change {
        n323 = event-data() -> ()  [unwired: 1 in, 6 out]
        n324 = call "set gain"("error in (no error)"=w539) -> ("gain"=w541:dbl, "OK"=w540:bool)  [unwired: 16 in, 1 out]
        n325 = case shown="True" w540 {
          tunnel: w541 -> [_ w542]
          frame False {
          }
          frame True {
            n326 = global write "GlobalSetGetConfigureCamera.vi" "gain"(w542) -> ()
          }
        }
      }
      event "Start": Value Change {
        n327 = event-data() -> ()  [unwired: 1 in, 6 out]
        n328 = global write "GetPicture.vi" "GetPicture"(TRUE ("GetPicture")) -> ()
      }
      event "Measurement Time": Value Change {
        n329 = event-data() -> ()  [unwired: 1 in, 6 out]
        n330 = global write "GlobalSetGetConfigureCamera.vi" "Exposure"(w544) -> ()
      }
      event "Stop": Value Change {
        n331 = event-data() -> ()  [unwired: 1 in, 6 out]
        n332 = global write "StopGetPic.vi" "Stop"(TRUE ("Stop")) -> ()
      }
      event "Stop Program": Value Change {
        n333 = event-data() -> ()  [unwired: 1 in, 6 out]
        n334 = flat-sequence {
          tunnel: w546 -> [w550]
          tunnel: [w550] -> w549
          frame #0 {
            n335 = local write "Global Stop"(TRUE ("Global Stop")) -> ()
          }
        }
        n336 = local read "PI SystemNumber"() -> (w548:i32)
        n337 = call "Close connection if open.vi"("System no."=w548, "error in"=w549) -> ("error out"=w547:errorcluster)  [unwired: 16 in, 1 out]
      }
    }
    "z-position" <- w103
    "y-position" <- w87
    "x-position" <- w102
  }
  n338 = while {
    shift-right: [w558] -> w10
    shift-left: w6 -> [w555]
    shift-right: [w560] -> _
    shift-left: w6 -> [w565]
    tunnel: w18 -> [w559]
    tunnel: "Image Measurent Parameters" -> [w554]
    tunnel: [w553] -> _
    tunnel: "Sample description" -> [w552]
    stop <- w563 stop-if-true
    n339 = case shown="No Error" w555 {
      selector: w555 -> [w571 w1441]
      tunnel: w565 -> [w581 w1443]
      tunnel: [w580 TRUE ("Global Stop")] -> w562
      tunnel: [w576 w1443] -> w561
      tunnel: w559 -> [w575 _]
      tunnel: [w574 w1441] -> w558
      tunnel: [w572 T25."No Measurement" ("Do Measurement")] -> w556
      tunnel: w554 -> [w569 _]
      tunnel: [w568 w1441] -> w553
      tunnel: w552 -> [w566 _]
      frame No Error {
        n340 = while {
          shift-right: [w1439] -> w577
          shift-left: w581 -> [w1439]
          tunnel: [w1434] -> w579
          tunnel: [w1436] -> w578
          tunnel: [w1435] -> w573
          stop <- w1440 stop-if-true
          w1435 = FALSE ("FiFo Overrun")
          # "Wait for Start"
          n341 = local read "Task"() -> (w1434:T10)
          n342 = local read "Global Stop"() -> (w1436:bool)
          n343 = Wait (ms)(milliseconds to wait=u32 100) -> ()  [unwired: 1 out]
          n344 = local write "Stop Measurement"(w1435) -> ()
          n345 = Greater Than 0?(x=w1434) -> (x > 0?=w1438:bool)
          n346 = Or(x=w1438, y=w1436) -> (x .or. y?=w1440:bool)
        }
        n347 = control-ref of="WS File Tree"() -> (w570:refnum<vi>)
        n348 = case shown="\"Save Color Image\"" w579 {
          selector: w579 -> [_ _ w947 _ _ _]
          tunnel: w571 -> [w582 w630 w855 w1129 w1198 w1397]
          tunnel: [w582 w600 w903 w1118 w1196 w1397] -> w574
          tunnel: [w583 FALSE ("Global Stop") FALSE ("Global Stop") FALSE ("Global Stop") FALSE ("Global Stop") FALSE ("Global Stop")] -> w580
          tunnel: w578 -> [w583 _ _ _ _ _]
          tunnel: w577 -> [w585 w614 w854 w1128 w1197 w1398]
          tunnel: [w585 w614 w968 w1128 w1197 w1396] -> w576
          tunnel: w575 -> [_ w680 w905 _ _ _]
          tunnel: [T25."No Measurement" ("Do Measurement") T25."No Measurement" ("Do Measurement") w946 T25."No Measurement" ("Do Measurement") T14."No Measurement" ("Do Measurement") w1395] -> w572
          tunnel: w570 -> [_ _ w936 _ _ _]
          tunnel: w569 -> [_ w658 _ _ _ _]
          tunnel: [w582 w632 w929 w1118 _ _] -> w568
          tunnel: "Laser pulse duration" -> [_ _ w911 _ _ _]
          tunnel: w566 -> [_ _ w902 _ _ _]
          frame "No Measurement", Default {
          }
          frame "Aquire Image" {
            w593 = 200
            w624 = T33."Image File" ("Measurement Type")
            w661 = 32768 ("dimension size")
            # "TODO:\n- FIFO Read Flag Buffer Half Full?\n- auto square pixels"
            # "Image Intensity Array"
            n349 = Index Array(array=w680) -> (element=w679:T34)  [unwired: 1 in]
            n350 = Unbundle By Name(w679) -> ("Dev"=w652:i32)
            n351 = local read "PI SystemNumber"() -> (w602:i32)
            n352 = Index Array(array=string[] ["yx", "yz", "xy", "xz", "zy", "zx"] ("Array"), index="Axis") -> (element=w607:string)
            n353 = stacked-sequence {
              seq-local: [w692 _] -> [_ w719]
              seq-local: [w691 _] -> [_ w720]
              seq-local: [w690 _] -> [_ w715]
              seq-local: [w686 _] -> [_ w713]
              seq-local: [w685 _] -> [_ w712]
              seq-local: [w684 _] -> [_ w711]
              seq-local: [w687 _] -> [_ w707]
              tunnel: "Picture size" -> [w705 _]
              tunnel: "Picture size 2" -> [w704 _]
              tunnel: w658 -> [w703 _]
              tunnel: "X-Position" -> [w702 _]
              tunnel: "Y-Position" -> [w701 _]
              tunnel: "Z-Position" -> [w700 _]
              tunnel: "Axis" -> [w694 _]
              tunnel: "Resolution" -> [w690 _]
              tunnel: [w693 _] -> w586
              tunnel: [_ w721] -> w631
              tunnel: w630 -> [w688 _]
              tunnel: w607 -> [_ w718]
              tunnel: "Laser  Profile" -> [_ w717]
              tunnel: "Pixel time" -> [w689 w716]
              tunnel: w602 -> [_ w714]
              tunnel: [_ w706] -> w627
              tunnel: [_ w710] -> w626
              tunnel: [_ w709] -> w625
              tunnel: [_ w708] -> w617
              frame #0 {
                n354 = call "PI_CheckScan.vi"("Picture size"=w705, "Picture size 2"=w704, "Axis"=w694, "x-Position"=w702, "y-Position"=w701, "z-Position"=w700, "error in (no error)"=w688) -> ("error out"=w687:errorcluster, "Picture size out"=w691:dbl, "Picture size out 2"=w692:dbl, "a0"=w686:dbl, "b0"=w685:dbl, "c0"=w684:dbl)  [unwired: 7 in]
                n355 = Divide(x=w691, y=w690) -> (x/y=w697:dbl)
                n356 = Divide(x=w692, y=w690) -> (x/y=w698:dbl)
                n357 = local write "Picture size 2"(w692) -> ()
                n358 = local write "Picture size"(w691) -> ()
                n359 = Round Toward +Infinity(x=w697) -> (ceil(x): smallest int >= x=w696:dbl)
                n360 = Round Toward +Infinity(x=w698) -> (ceil(x): smallest int >= x=w695:dbl)
                n361 = Bundle("a0"=w686, "b0"=w685, "c0"=w684) -> (w699:cluster{"a0":dbl, "b0":dbl, "c0":dbl})  [unwired: 1 in]
                n362 = Bundle By Name(cluster=w703, "Position"=w699, "Axis 1 Pixels"=w696, "Axis 2 Pixels"=w695, "Axis"=w694, "Resolution"=w690, "PixelTime"=w689) -> (w693:T8)
              }
              frame #1 {
                n363 = call "PI_AreaScan_Prepare_1.vi"("System"=w714, "Laser"=w717, "Axis"=w718, "da"=w720, "db"=w719, "error in (no error)"=w707, "a0"=w713, "b0"=w712, "Resolution"=w715, "c0"=w711, "Pixel time"=w716) -> ("Tacq"=w706:dbl, "lp"=w709:i32, "ap"=w710:i32, "Trigger"=w708:dbl[], "error out"=w721:errorcluster)  [unwired: 4 in]
                "Measure. time" <- w706
              }
            }
            n364 = String To Byte Array(string="Laser  Profile") -> (unsigned byte array=w609:u8[])
            n365 = Unbundle By Name(w586) -> ("Axis 1 Pixels"=w639:dbl, "Axis 2 Pixels"=w640:dbl, "Resolution"=w637:dbl, "PixelTime"=w621:dbl)  [unwired: 2 out]
            n366 = control-ref of="WS File Tree"() -> (w664:refnum<vi>)
            n367 = local read "Workspace"() -> (w669:path)
            n368 = Divide(x=w639, y=w637) -> (x/y=w648:dbl)
            n369 = Divide(x=w640, y=w637) -> (x/y=w650:dbl)
            n370 = call "HH_Set.vi"("Device List"=w680, "CFD Settings"="CFD Settings", "error in (no error)"=w631, "SyncDiv"=8) -> ("ht3 header out"=w644:T35, "Sync Rate"=w642:i32, "error out"=w616:errorcluster)  [unwired: 7 in, 2 out]
            n371 = Divide(x=w621, y=1000) -> (x/y=w619:dbl)
            n372 = control-ref of="Image"() -> (w646:refnum<vi>)
            n373 = Round Toward +Infinity(x=w648) -> (ceil(x): smallest int >= x=w647:dbl)
            n374 = Round Toward +Infinity(x=w650) -> (ceil(x): smallest int >= x=w649:dbl)
            n375 = call "MTS_PreapareImage.vi"("WS File Tree"=w664, "Workspace"=w669, "Measurement Type"=w624, "Image Measurent Parameters"=w586, "error in"=w616, "Trigger"=w617) -> ("File Name (dup)"=w654:path, "File No"=→"Last Image File No":i32, "Image Header"=w656:T36, "Comment"=w657:string, "error out"=w615:errorcluster)  [unwired: 5 in]
            n376 = Divide(x=1024, y=w642) -> (x/y=w623:dbl)
            n377 = local write "Active pt3"(w654) -> ()
            n378 = Multiply(x=w627, y=1000) -> (x*y=w636:dbl)
            n379 = call "Scan_SetGraphScales.vi"("error in (no error)"=w615, "Image Measurent Parameters"=w586, "Image"=w646) -> ("error out"=w645:errorcluster)  [unwired: 8 in]
            n380 = Subtract(x=w609, y=48) -> (x-y=w608:i32[])
            n381 = Initialize Array(0 ("element"), w647, w649) -> (w620:i32[][])
            n382 = Initialize Array(0, 5, 2) -> (w606:i32[][])
            n383 = Replace Array Subset(array=w606, new element=w608, index (col)=0) -> (w604:i32[][])  [unwired: 1 in]
            n384 = call "HT3_Create.vi"("Laser"=w604, "Image Header in"=w656, "Save pt3"="Save Files", "Measurement Type"=w624, "error in"=w645, "Comment"=w657, "ht3 Header in"=w644, "File Path"=w654) -> ("error out"=w670:errorcluster, "FileHeaderPos"=w660:T37, "refnum out"=w668:refnum<file>)  [unwired: 1 in]
            n385 = Round Toward +Infinity(x=w636) -> (ceil(x): smallest int >= x=w634:dbl)
            n386 = call "HH_Start.vi"("Device Index"=w652, "Acq. Time"=w634, "error in (no error)"=w670) -> ("error out"=w677:errorcluster)  [unwired: 11 in, 1 out]
            n387 = Unbundle By Name(w677) -> ("status"=w678:bool)
            n388 = Not(x=w678) -> (.not. x?=w676:bool)
            n389 = Initialize Array(u32 0, w661) -> (w673:u32[])
            n390 = case shown="True" w676 {
              tunnel: [w769 w800] -> w675
              tunnel: w602 -> [_ w795]
              tunnel: w677 -> [w770 w796]
              tunnel: w652 -> [w768 w787]
              tunnel: w620 -> [_ w772]
              tunnel: w673 -> [_ w794]
              tunnel: w661 -> [_ w793]
              tunnel: [w767 w792] -> w672
              tunnel: [w767 w791] -> w671
              tunnel: w668 -> [w766 w790]
              tunnel: [w766 w789] -> w667
              tunnel: [0 ("Num Records Total") w788] -> w666
              tunnel: [0.0 w781] -> w665
              tunnel: w607 -> [_ w784]
              tunnel: [dbl[] [] w778] -> w622
              tunnel: w619 -> [_ w774]
              tunnel: w617 -> [_ w773]
              frame False {
                (unwired) i32[][] [] ("Image Array Out")
                (unwired) u64[] [] ("Histograms")
                w767 = FALSE ("Stop Measurement")
                n391 = call "HH_Stop.vi"("Device Index"=w768, "error in (no error)"=w770) -> ("error out"=w769:errorcluster)  [unwired: 12 in, 1 out]
              }
              frame True {
                # "Overflow Interv. Time (s)"
                # "No Error"
                n392 = call "PI Start WG.vi"("System no."=w795, "axis"=w784, "Generator"=T26."both axis", "Init DDL"=T27."none", "increment"=T27."slow axis", "error in"=w796, "saved data"=T28."actual position") -> ("error out"=w797:errorcluster)  [unwired: 12 in]
                n393 = Initialize Array(0, 5) -> (w775:i32[])
                n394 = while {
                  tunnel: w787 -> [w820]
                  tunnel: w794 -> [w836]
                  tunnel: w793 -> [w835]
                  shift-right: [w821] -> w799
                  shift-left: w797 -> [w837]
                  shift-right: [FALSE ("Reset")] -> _
                  shift-left: TRUE ("Reset") -> [w808]
                  tunnel: [w829] -> w792
                  tunnel: [w825] -> w791
                  tunnel: w790 -> [w827]
                  tunnel: [w826] -> w789
                  tunnel: [w804] -> w788
                  tunnel: [w803] -> w781
                  shift-right: [w817] -> w780
                  shift-left: w775 -> [w815]
                  tunnel: [w814] -> w779
                  tunnel: w774 -> [w811]
                  tunnel: w773 -> [_]
                  shift-right: [w802] -> w771
                  shift-left: w772 -> [w810]
                  i -> [w813]
                  stop <- w834 stop-if-true
                  n395 = call "HH_FIFORead.vi"("Device Index"=w820, "Buffer In"=w836, "Count"=w835, "error in (no error)"=w837) -> ("OK"=w830:bool, "Buffer Out"=w807:u32[], "Data Count"=w806:i32, "FiFo Overrun"=w829:bool, "error out"=w828:errorcluster)  [unwired: 7 in]
                  n396 = local write "Buffer Overrun"(w829) -> ()
                  n397 = Unbundle(w828) -> ("status"=w833:bool)  [unwired: 2 out]
                  n398 = call "HT3_Write.vi"("error in"=w828, "Data Count"=w806, "Data in"=w807, "refnum in"=w827) -> ("error out"=w822:errorcluster, "refnum out"=w826:refnum<file>)  [unwired: 6 in]
                  n399 = call "GetCountRates.vi"("error in (no error)"=w822, "DeviceIndex"=w820) -> ("error out"=w821:errorcluster, "CntRates"=w819:dbl[], "SyncRate"=w812:i32)  [unwired: 1 in]
                  n400 = local read "Stop Measurement"() -> (w824:bool)
                  n401 = local read "Global Stop"() -> (w823:bool)
                  n402 = Multiply(x=w811, y=w812) -> (x*y=w801:dbl)
                  n403 = Compound Arithmetic op=OR(invert w830, w833, w823, w824) -> (w834:bool)
                  n404 = Insert Into Array(array=w819, index=0, new element=w812) -> (w816:dbl[])
                  n405 = call "HH_ToImage.vi"("Data In"=w807, "Reset"=w808, "Image Array In"=w810, "Data Count"=w806, "Pixel Time (Laser Pulses)"=w801) -> ("Image Array Out"=w802:i32[][], "Histograms"=→"Histogram":i32[][], "Total Oveflow Count"=w803:u64, "Num Records Total"=w804:i64, "Traces"=→"Trace":i32[][])  [unwired: 4 in, 2 out]
                  n406 = Or(x=w824, y=w823) -> (x .or. y?=w825:bool)
                  n407 = Add(x=w815, y=w816) -> (x+y=w817:dbl[])
                  n408 = Wait (ms)(milliseconds to wait=u32 2) -> ()  [unwired: 1 out]
                  n409 = Increment(x=w813) -> (x+1=w814:i32)
                }
                "Image" <- w771
                n410 = call "HH_Stop.vi"("Device Index"=w787, "error in (no error)"=w799) -> ("error out"=w800:errorcluster)  [unwired: 12 in, 1 out]
                n411 = Divide(x=w780, y=w779) -> (x/y=w778:dbl[])
              }
            }
            n412 = flat-sequence {
              tunnel: w675 -> [w740]
              tunnel: [w729] -> w601
              tunnel: w672 -> [w742]
              tunnel: w671 -> [w731]
              tunnel: w602 -> [w739]
              tunnel: [w738] -> w599
              tunnel: w667 -> [w736]
              tunnel: w666 -> [w735]
              tunnel: w665 -> [w725]
              tunnel: w660 -> [w730]
              tunnel: w623 -> [w726]
              tunnel: w622 -> [w722]
              frame #0 {
                # "Count Rate (per s)"
                # "Finish after Aquire Image"
                n413 = Multiply(x=w726, y=w725) -> (x*y=w724:dbl)
                n414 = Or(x=w731, y=w742) -> (x .or. y?=w741:bool)
                n415 = case shown="False" w741 {
                  tunnel: w740 -> [w747 w757]
                  tunnel: w739 -> [w745 w758]
                  tunnel: [w744 w758] -> w738
                  tunnel: [w746 w756] -> w737
                  tunnel: [enum16{"timeover", "manual", "overflow"}."timeover" ("Stop Reason") w761] -> w732
                  tunnel: w731 -> [w743 w759]
                  frame False {
                    # "Stop WaveGen\nif Aborted"
                    n416 = case shown="True" w743 {
                      tunnel: w747 -> [w749 w754]
                      tunnel: [w749 w753] -> w746
                      tunnel: w745 -> [w750 w752]
                      tunnel: [w750 w752] -> w744
                      frame False {
                      }
                      frame True {
                        n417 = call "PI Write GPIB.vi"("System no."=w752, "String to send"="0RT", "error in"=w754) -> ("error out"=w753:errorcluster)  [unwired: 16 in]
                      }
                    }
                  }
                  frame True {
                    n418 = Select(t=enum16{"timeover", "manual", "overflow"}."manual" ("Stop Reason"), s=w759, f=enum16{"timeover", "manual", "overflow"}."overflow" ("Stop Reason")) -> (s? t:f=w761:enum16{"timeover", "manual", "overflow"})
                    n419 = call "PI Write GPIB.vi"("System no."=w758, "String to send"="0RT", "error in"=w757) -> ("error out"=w756:errorcluster)  [unwired: 16 in]
                  }
                }
                n420 = Multiply(x=w724, y=1000.0) -> (x*y=w734:dbl)
                n421 = property on="Aquire Image" class="Bool"("BoolText.Text"="Aquire Image" ("Caption.Text"), "BoolText.TextColor"=u32 0 ("Boolean Text.Colors:FG Color")) -> ()  [unwired: 2 in, 2 out]
                n422 = To Long Integer(number=w734) -> (32bit integer=w733:i32)
                n423 = call "HT3_Finish.vi"("FileHeaderPos"=w730, "Rates"=w722, "Stop Reason"=w732, "error in"=w737, "Num Records"=w735, "Stop After (ms)"=w733, "refnum in"=w736) -> ("error out"=w729:errorcluster)  [unwired: 4 in]
              }
            }
            n424 = local read "X-Position"() -> (w592:dbl)
            n425 = local read "Y-Position"() -> (w591:dbl)
            n426 = local read "Z-Position"() -> (w590:dbl)
            n427 = Subtract(x=w593, y=w592) -> (x-y=w589:dbl)
            n428 = Subtract(x=w593, y=w591) -> (x-y=w588:dbl)
            n429 = Subtract(x=w593, y=w590) -> (x-y=w587:dbl)
            n430 = global read "GlobalConAxisPI.vi" "Conn. Axes"() -> (w598:string[])
            n431 = call "AOTF-Trigger_1.vi"("Channel"="Laser  Profile", "error in (no error)"=w631, "Triggered"=TRUE, "lp"=w625, "ap"=w626) -> ("error out"=w632:errorcluster)  [unwired: 2 in]
            n432 = Build Array(w589, w588, w587) -> (w597:dbl[])
            n433 = call "MOV.vi"("System no."=w599, "Axes to move"=w598, "Position values"=w597, "error in"=w601) -> ("error out"=w600:errorcluster)  [unwired: 15 in]
          }
          frame "Point Measurement", "Auto Point" {
            w873 = 200
            w878 = 200
            w906 = 0
            w934 = 32768 ("dimension size")
            n434 = Index Array(array=w905) -> (element=w972:T34)  [unwired: 1 in]
            n435 = Unbundle By Name(w972) -> ("Dev"=w891:i32)
            n436 = Equal?(x=w947, y=T10."Auto Point" ("Task")) -> (x = y?=w843:bool)
            n437 = local read "concatenated string"() -> (w898:string)
            n438 = And(x=w843, y="Autopoint-Autofocus Z") -> (x .and. y?=w935:bool)
            n439 = Or(x="Point Defocussed Cam", y="Auto Defocussed Cam") -> (x .or. y?=w860:bool)
            n440 = Select(t="Auto Measurement Time (ms)", s=w843, f="Measurement Time") -> (s? t:f=w844:i32)
            n441 = local read "X-Position"() -> (w953:dbl)
            n442 = local read "Y-Position"() -> (w952:dbl)
            n443 = local read "Z-Position"() -> (w888:dbl)
            n444 = Select(t="AutoPoint" ("Measurement Type"), s=w843, f="Point" ("Measurement Type")) -> (s? t:f=w897:string)
            n445 = case shown="True" w860 {
              tunnel: [w974 w979] -> w853
              tunnel: w854 -> [w974 w980]
              tunnel: w844 -> [_ w977]
              frame False {
              }
              frame True {
                n446 = global read "GlobalSetGetConfigureCamera.vi" "Exposure"() -> (w975:sgl)
                n447 = Greater?(x=w975, y=w977) -> (0:w978:bool)
                n448 = case shown="False" w978 {
                  tunnel: w977 -> [_ w982]
                  tunnel: [w981 w982] -> w976
                  tunnel: w975 -> [w981 _]
                  frame False {
                  }
                  frame True {
                  }
                }
                n449 = call "PrepCamera.vi"("mesTime"=w976, "error out 2"=w980) -> ("error out"=w979:errorcluster)  [unwired: 25 in]
              }
            }
            n450 = Select(t=T10."Auto Measurement Control" ("Task"), s=w843, f=T25."No Measurement" ("Do Measurement")) -> (s? t:f=w946:T10)
            n451 = local read "NxtAutMesPoint"() -> (w892:i32)
            n452 = Multiply(x=w844, y=1000) -> (x*y=w845:i32)
            n453 = local read "Pattern"() -> (w893:dbl[][])
            n454 = Concatenate Strings(w898, w897) -> (w896:string)
            n455 = Bundle("X-Position"=w953, "Y-Position"=w952, "Z-Position"=w888) -> (w937:T38)  [unwired: 1 in]
            n456 = call "MTS_AutoPointCords.vi"("Is Auto Point"=w843, "Cords In"=w937, "Next Auto Measure Point"=w892, "Pattern"=w893) -> ("Cords"=w924:T38)  [unwired: 7 in]
            n457 = Unbundle By Name(w924) -> ("X-Position"=w864:dbl, "Y-Position"=w865:dbl, "Z-Position"=w874:dbl)
            n458 = Subtract(x=w878, y=w865) -> (x-y=w877:dbl)
            n459 = Subtract(x=w878, y=w864) -> (x-y=w876:dbl)
            n460 = Subtract(x=w878, y=w874) -> (x-y=w875:dbl)
            n461 = local read "PI SystemNumber"() -> (w886:i32)
            n462 = global read "GlobalConAxisPI.vi" "Conn. Axes"() -> (w880:string[])
            n463 = Build Array(w877, w876, w875) -> (w879:dbl[])
            n464 = local read "Last Image File No"() -> (w940:i32)
            n465 = call "MOV.vi"("System no."=w886, "Axes to move"=w880, "Position values"=w879, "No.of digits"=i16 3, "error in"=w855) -> ("error out"=w868:errorcluster)  [unwired: 14 in]
            n466 = flat-sequence {
              tunnel: w868 -> [w983]
              tunnel: [w983] -> w867
              frame #0 {
                n467 = Wait (ms)(milliseconds to wait=u32 100) -> ()  [unwired: 1 out]
              }
            }
            n468 = Select(t=T29."Auto Point" ("Measurement Type"), s=w843, f=T29."Point Measurement" ("Measurement Type")) -> (s? t:f=w941:T29)
            n469 = Select(t=w940, s=w843, f=-1) -> (s? t:f=w938:i32)
            n470 = local read "Workspace"() -> (w962:path)
            n471 = call "MTS_GenFileComment.vi"("Measurement Type"=w941, "Parent File No"=w938, "Info"=w902, "Upper Left"=w924, "error in"=w853) -> ("Comment"=w963:string, "error out"=w961:errorcluster)  [unwired: 7 in, 2 out]
            n472 = Not(x="Adjustment") -> (.not. x?=w900:bool)
            n473 = call "MTS_GetNextFileName.vi"("error in (no error)"=w961, "File Type"="ht3", "Measurement Type"=w896, "Workspace"=w962) -> ("error out"=w956:errorcluster, "Next File Name"=w955:path)  [unwired: 6 in]
            n474 = local read "CFD Settings"() -> (w931:T7)
            n475 = case shown="True" w900 {
              tunnel: w956 -> [w997 w1005]
              tunnel: w955 -> [_ w1004]
              tunnel: [w997 w1003] -> w856
              tunnel: [path "D:/tmp.ht3" w998] -> w954
              tunnel: w941 -> [_ w1000]
              tunnel: w938 -> [_ w1002]
              tunnel: w936 -> [_ w999]
              frame False {
              }
              frame True {
                n476 = call "MTS_AddFileToWorkspace.vi"("File Name"=w1004, "File Type"=T30."pt3 File", "Measurement Type"=w1000, "error in (no error)"=w1005, "Parent"=w1002, "Tree Refnum"=w999) -> ("File Name (dup)"=w998:path, "error out"=w1003:errorcluster)  [unwired: 7 in, 1 out]
              }
            }
            n477 = call "POS?.vi"("System no."=w886, "Axes to query"=w880, "All axes?"=TRUE, "error in"=w867) -> ("Position"=w884:dbl[], "error out"=w887:errorcluster)  [unwired: 14 in]
            n478 = call "HH_Set.vi"("Device List"=w905, "CFD Settings"=w931, "error in (no error)"=w887) -> ("ht3 header out"=w951:T35, "Sync Rate"=w921:i32, "error out"=w949:errorcluster)  [unwired: 8 in, 2 out]
            n479 = Index Array(array=w884, index #1=0 ("index"), index #2=1 ("index"), index #3=2 ("index")) -> (element #1=w872:dbl, element #2=w871:dbl, element #3=w870:dbl)
            n480 = Bundle By Name(cluster=w951, "AcquisitionTime (ms)"=w845) -> (w950:T35)
            n481 = Divide(x=65536 ("n"), y=w921) -> (x/y=w922:dbl)
            n482 = Subtract(x=w873, y=w872) -> (x-y=w842:dbl)
            n483 = Subtract(x=w873, y=w870) -> (x-y=w869:dbl)
            n484 = Subtract(x=w873, y=w871) -> (x-y=w841:dbl)
            n485 = property on="y-position" class="DigNum (strict)"("Value"=w842) -> ()  [unwired: 2 in, 2 out]
            n486 = property on="z-position" class="DigNum (strict)"("Value"=w869) -> ()  [unwired: 2 in, 2 out]
            n487 = case shown="True" w935 {
              tunnel: w949 -> [w1006 w1014]
              tunnel: [w1006 w1013] -> w948
              tunnel: w886 -> [_ w1008]
              tunnel: w922 -> [_ w1012]
              tunnel: w924 -> [_ w1011]
              tunnel: w891 -> [_ w1007]
              frame False {
              }
              frame True {
                # "Auto Z"
                n488 = call "MTS_AutoZPos.vi"("PH Dev"=w1007, "OFlow Interv [s]"=w1012, "PI System no."=w1008, "error in"=w1014, "Start Point"=w1011) -> ("New Z"=w1010:dbl, "Counts"=→"Counts":u32[], "error out"=w1013:errorcluster)  [unwired: 7 in, 1 out]
                n489 = local write "Z-Position"(w1010) -> ()
              }
            }
            n490 = property on="x-position" class="DigNum (strict)"("Value"=w841) -> ()  [unwired: 2 in, 2 out]
            n491 = Initialize Array(u32 0, w934) -> (w966:u32[])
            n492 = global read "ccdChipPixels.vi" "CCD Chip horizontal start"() -> (w851:i32)
            n493 = global read "ccdChipPixels.vi" "CCD Chip horizontal end"() -> (w852:i32)
            n494 = global read "ccdChipPixels.vi" "CCD Chip Vertical Start"() -> (w849:i32)
            n495 = global read "ccdChipPixels.vi" "CCD Chip Vertical end"() -> (w850:i32)
            n496 = Subtract(x=w852, y=w851) -> (x-y=w847:i32)
            n497 = Subtract(x=w850, y=w849) -> (x-y=w846:i32)
            n498 = flat-sequence {
              tunnel: w969 -> [w1018]
              tunnel: w857 -> [w1035]
              tunnel: [w1016] -> w968
              tunnel: [w1032] -> w904
              tunnel: w965 -> [w1037]
              tunnel: w964 -> [w1028]
              tunnel: w958 -> [w1031]
              tunnel: w957 -> [w1030]
              tunnel: w933 -> [w1027]
              tunnel: w926 -> [w1024]
              tunnel: w925 -> [w1023]
              tunnel: w860 -> [w1015]
              frame #0 {
                # "Finish after Measurement"
                n499 = case shown="False" w1015 {
                  tunnel: w1018 -> [w1039 w1044]
                  tunnel: [w1039 w1041] -> w1017
                  frame False {
                  }
                  frame True {
                    n500 = call "SetShutter.vi"("type"=Shutter_type_typedef."TTL High", "mode"=Shutter_mode_typedef."Close", "error in (no error)"=w1044) -> ("error out"=w1046:errorcluster)  [unwired: 11 in, 1 out]
                    n501 = call <vilib>:"Clear Errors.vi"("error in (no error)"=w1046) -> ("error out"=w1045:errorcluster)  [unwired: 6 in]
                    n502 = call "AbortAcquisition.vi"("error in (no error)"=w1045) -> ("error out"=w1040:errorcluster)  [unwired: 1 in, 1 out]
                    n503 = call <vilib>:"Clear Errors.vi"("error in (no error)"=w1040) -> ("error out"=w1041:errorcluster)  [unwired: 6 in]
                  }
                }
                n504 = Or(x=w1028, y=w1037) -> (x .or. y?=w1036:bool)
                n505 = Index Array(array=w1024, index=0) -> (element=w1025:dbl)
                n506 = case shown="False" w1036 {
                  tunnel: w1035 -> [w1048 w1049]
                  tunnel: [w1048 w1049] -> w1033
                  tunnel: [enum16{"timeover", "manual", "overflow"}."timeover" ("Stop Reason") w1052] -> w1029
                  tunnel: w1028 -> [_ w1050]
                  frame False {
                  }
                  frame True {
                    n507 = Select(t=enum16{"timeover", "manual", "overflow"}."manual" ("Stop Reason"), s=w1050, f=enum16{"timeover", "manual", "overflow"}."overflow" ("Stop Reason")) -> (s? t:f=w1052:enum16{"timeover", "manual", "overflow"})
                  }
                }
                n508 = Divide(x=w1023, y=w1025) -> (x/y=w1022:dbl)
                n509 = Multiply(x=1024000, y=w1022) -> (x*y=w1020:dbl)
                n510 = To Long Integer(number=w1020) -> (32bit integer=w1019:i32)
                n511 = property on="Point Measurement" class="Bool"("BoolText.Text"="Point Measurement" ("Caption.Text"), "BoolText.TextColor"=u32 0 ("Boolean Text.Colors:FG Color")) -> ()  [unwired: 2 in, 2 out]
                n512 = call "HT3_Finish.vi"("FileHeaderPos"=w1027, "Rates"=w1024, "Stop Reason"=w1029, "error in"=w1033, "Num Records"=w1030, "Stop After (ms)"=w1019, "refnum in"=w1031) -> ("error out"=w1032:errorcluster)  [unwired: 4 in]
                n513 = Merge Errors(w1018, w1017) -> (w1016:errorcluster)
              }
            }
            n514 = local read "Laser  Profile"() -> (w920:string)
            n515 = String To Byte Array(string=w920) -> (unsigned byte array=w918:u8[])
            n516 = Subtract(x=w918, y=48) -> (x-y=w913:i32[])
            n517 = String Length(string=w920) -> (length=w910:i32)
            n518 = Initialize Array(0, 5, 2) -> (w914:i32[][])
            n519 = Replace Array Subset(array=w914, new element=w913, index (col)=w906) -> (w912:i32[][])  [unwired: 1 in]
            n520 = Array Subset(array=w911, index=w906, length=w910) -> (w909:i32[])
            n521 = Replace Array Subset(array=w912, new element=w909, index (col)=1) -> (w908:i32[][])  [unwired: 1 in]
            n522 = call "HT3_Create.vi"("Laser"=w908, "Save pt3"=w900, "error in"=w948, "Comment"=w963, "ht3 Header in"=w950, "File Path"=w954) -> ("error out"=w889:errorcluster, "FileHeaderPos"=w933:T37, "refnum out"=w959:refnum<file>)  [unwired: 3 in]
            n523 = call "HH_Start.vi"("Device Index"=w891, "Acq. Time"=w845, "error in (no error)"=w889) -> ("error out"=w859:errorcluster)  [unwired: 11 in, 1 out]
            n524 = case shown="True" w860 {
              tunnel: [w985 w989] -> w839
              tunnel: w889 -> [w985 w988]
              tunnel: w843 -> [_ w987]
              tunnel: [_ w986] -> w848
              frame False {
              }
              frame True {
                n525 = control-ref of="NxtAutMesPoint"() -> (w994:refnum<vi>)
                n526 = control-ref of="Workspace"() -> (w995:refnum<vi>)
                n527 = control-ref of="y-position"() -> (w991:refnum<vi>)
                n528 = control-ref of="x-position"() -> (w992:refnum<vi>)
                n529 = control-ref of="z-position"() -> (w990:refnum<vi>)
                n530 = control-ref of="Pattern"() -> (w993:refnum<vi>)
                n531 = call "DefocussedImage.vi"("Path in"=w995, "reference"=w994, "Boolean"=w987, "reference 2"=w993, "reference 3"=w992, "error in (no error)"=w988, "reference 4"=w991, "reference 5"=w990) -> ("camout"=w986:i32[], "error out"=w989:errorcluster)  [unwired: 6 in]
              }
            }
            n532 = Unbundle By Name(w859) -> ("status"=w971:bool)
            n533 = Not(x=w971) -> (.not. x?=w970:bool)
            n534 = case shown="True" w970 {
              tunnel: [w1060 w1063] -> w858
              tunnel: w859 -> [w1061 w1072]
              tunnel: w856 -> [w1062 w1083]
              tunnel: [w1062 w1082] -> w969
              tunnel: w891 -> [w1055 w1071]
              tunnel: w966 -> [_ w1079]
              tunnel: w934 -> [_ w1078]
              tunnel: [w1059 w1077] -> w965
              tunnel: [w1059 w1076] -> w964
              tunnel: w959 -> [w1058 w1075]
              tunnel: [w1058 w1074] -> w958
              tunnel: [i64 0 ("Num Records Total") w1073] -> w957
              tunnel: [dbl[] [] w1068] -> w926
              tunnel: [0 w1067] -> w925
              frame False {
                w1059 = FALSE ("Stop Measurement")
                n535 = call "HH_Stop.vi"("Device Index"=w1055, "error in (no error)"=w1061) -> ("error out"=w1060:errorcluster)  [unwired: 12 in, 1 out]
              }
              frame True {
                # "Overflow Interv. Time (s)"
                # "No Error"
                n536 = Initialize Array(0, 5) -> (w1066:i32[])
                n537 = while {
                  tunnel: w1071 -> [w1092]
                  tunnel: w1079 -> [w1116]
                  tunnel: w1078 -> [w1115]
                  shift-right: [w1093] -> w1081
                  shift-left: w1072 -> [w1117]
                  shift-right: [w1114] -> w1082
                  shift-left: w1083 -> [w1114]
                  shift-right: [FALSE ("Reset")] -> _
                  shift-left: TRUE ("Reset") -> [w1110]
                  tunnel: [w1107] -> w1077
                  tunnel: [w1099] -> w1076
                  tunnel: w1075 -> [w1103]
                  tunnel: [w1102] -> w1074
                  tunnel: [w1101] -> w1073
                  tunnel: [w1100] -> w1067
                  shift-right: [w1087] -> w1069
                  shift-left: w1066 -> [w1086]
                  tunnel: [w1084] -> w1070
                  i -> [w1085]
                  stop <- w1113 stop-if-true
                  n538 = call "HH_FIFORead.vi"("Device Index"=w1092, "Buffer In"=w1116, "Count"=w1115, "error in (no error)"=w1117) -> ("OK"=w1108:bool, "Buffer Out"=w1104:u32[], "Data Count"=w1105:i32, "FiFo Overrun"=w1107:bool, "error out"=w1106:errorcluster)  [unwired: 7 in]
                  n539 = Wait (ms)(milliseconds to wait=u32 10) -> ()  [unwired: 1 out]
                  n540 = local write "Buffer Overrun"(w1107) -> ()
                  n541 = Unbundle(w1106) -> ("status"=w1112:bool)  [unwired: 2 out]
                  n542 = call "HT3_Write.vi"("error in"=w1106, "Data Count"=w1105, "Data in"=w1104, "refnum in"=w1103) -> ("error out"=w1094:errorcluster, "refnum out"=w1102:refnum<file>)  [unwired: 6 in]
                  n543 = call "HH_TraceAndHisto.vi"("Data In"=w1104, "Reset"=w1110, "Data Count"=w1105) -> ("Histograms"=w1096:i32[][], "Total Oveflow Count"=w1100:u64, "Num Records Total"=w1101:i64, "Traces"=w1095:i32[][])  [unwired: 8 in, 1 out]
                  n544 = local read "Stop Measurement"() -> (w1098:bool)
                  n545 = local read "Global Stop"() -> (w1097:bool)
                  n546 = local write "Trace"(w1095) -> ()
                  n547 = call "GetCountRates.vi"("error in (no error)"=w1094, "DeviceIndex"=w1092) -> ("error out"=w1093:errorcluster, "CntRates"=w1088:dbl[], "SyncRate"=w1089:i32)  [unwired: 1 in]
                  n548 = local write "Histogram"(w1096) -> ()
                  n549 = Compound Arithmetic op=OR(invert w1108, w1112, w1097, w1098) -> (w1113:bool)
                  n550 = Insert Into Array(array=w1088, index=0, new element=w1089) -> (w1090:dbl[])
                  n551 = Or(x=w1098, y=w1097) -> (x .or. y?=w1099:bool)
                  n552 = Add(x=w1086, y=w1090) -> (x+y=w1087:dbl[])
                  n553 = Increment(x=w1085) -> (x+1=w1084:i32)
                }
                n554 = Divide(x=w1069, y=w1070) -> (x/y=w1068:dbl[])
                n555 = call "HH_Stop.vi"("Device Index"=w1071, "error in (no error)"=w1081) -> ("error out"=w1063:errorcluster)  [unwired: 12 in, 1 out]
              }
            }
            n556 = Reshape Array(w848, w847, w846) -> (w840:i32[][])
            n557 = property on="Point" class="IntGraph (strict)"(error in=w839, "Value"=w840) -> (error out=w838:errorcluster)  [unwired: 1 in, 1 out]
            n558 = Merge Errors(w858, w838) -> (w857:errorcluster)
            n559 = call "AOTF-Trigger_1.vi"("Channel"=w920, "Pulse length"=w911, "Sync trigger ratio"=5, "error in (no error)"=w855, "Triggered"=FALSE) -> ("error out"=w929:errorcluster)  [unwired: 2 in]
            n560 = call "MOV.vi"("System no."=w886, "Axes to move"=w880, "Position values"=w879, "error in"=w904) -> ("error out"=w903:errorcluster)  [unwired: 15 in]
          }
          frame "Save Color Image" {
            n561 = local read "Active pt3"() -> (w1125:path)
            n562 = call "MTS_GetFileFromWS.vi"(".pt3 File Name"=w1125) -> ("File Header"=w1124:T39)  [unwired: 9 in, 1 out]
            n563 = Unbundle By Name(w1124) -> ("Measurement Type"=w1123:T40, "Pixels"=w1120:i32[])
            n564 = control-ref of="WS File Tree"() -> (w1126:refnum<vi>)
            n565 = Equal?(x=T29."Image File" ("Measurement Type"), y=w1123) -> (x = y?=w1121:bool)
            n566 = case shown="True" w1121 {
              tunnel: w1129 -> [w1130 w1153]
              tunnel: w1125 -> [_ w1152]
              tunnel: w1125 -> [_ _]
              tunnel: [w1130 w1132] -> w1118
              tunnel: w1126 -> [_ _]
              tunnel: w1120 -> [_ w1137]
              frame False {
              }
              frame True {
                # "Image Intensity Array"
                # "Image Intensity Array"
                n567 = call "HT3_Open.vi"("error in"=w1153, "File Path"=w1152) -> ("error out"=w1145:errorcluster, "Header"=w1149:T41, "refnum out"=w1151:refnum<file>)  [unwired: 3 in, 4 out]
                n568 = Unbundle By Name(w1149) -> ()  [unwired: 15 out]
                n569 = Index Array(array=w1137, index #2=1 ("index")) -> (element #1=w1134:i32, element #2=w1135:i32)  [unwired: 1 in]
                n570 = Initialize Array(0 ("element"), w1134, w1135) -> (w1147:i32[][])
                n571 = Initialize Array(0 ("element"), 4 ("dimension size"), w1134, w1135) -> (w1140:i32[][][])
                n572 = while {
                  tunnel: w1151 -> [w1178]
                  shift-right: [FALSE ("Start From Top")] -> _
                  shift-left: TRUE ("Start From Top") -> [w1172]
                  shift-right: [w1171] -> w1144
                  shift-left: w1145 -> [w1169]
                  tunnel: [w1170] -> w1143
                  tunnel: w1147 -> [w1168]
                  tunnel: [w1167] -> w1146
                  tunnel: [w1168] -> _
                  stop <- w1175 stop-if-true
                  n573 = call "HT3_Read.vi"("Start From Top"=w1172, "error in"=w1169, "Data count"=10000, "refnum in"=w1178) -> ("error out"=w1171:errorcluster, "Data out"=w1174:u32[], "refnum out"=w1170:refnum<file>, "EOF?"=w1175:bool)  [unwired: 4 in]
                  n574 = Array Size(array=w1174) -> (size(s)=w1173:i32)
                  n575 = call "HH_FileToImage_1.vi"("Data In"=w1174, "Reset"=w1172, "Data Count"=w1173) -> ("Histograms"=w1167:i32[][])  [unwired: 7 in, 5 out]
                }
                n576 = call "MTS_SelectTCSPCBinning.vi"("Histograms in"=w1146) -> ("TCSPC Binning"=w1139:i32[][])  [unwired: 1 in, 9 out]
                n577 = while {
                  tunnel: w1143 -> [w1166]
                  shift-right: [FALSE ("Start From Top")] -> _
                  shift-left: TRUE ("Start From Top") -> [w1160]
                  shift-right: [w1159] -> w1131
                  shift-left: w1144 -> [w1155]
                  tunnel: [w1158] -> w1133
                  tunnel: w1140 -> [w1157]
                  tunnel: [w1156] -> _
                  tunnel: w1139 -> [w1154]
                  stop <- w1163 stop-if-true
                  n578 = call "HT3_Read.vi"("Start From Top"=w1160, "error in"=w1155, "Data count"=10000, "refnum in"=w1166) -> ("error out"=w1159:errorcluster, "Data out"=w1162:u32[], "refnum out"=w1158:refnum<file>, "EOF?"=w1163:bool)  [unwired: 4 out]
                  n579 = Array Size(array=w1162) -> (size(s)=w1161:i32)
                  n580 = call "HH_ToColorImage.vi"("Data In"=w1162, "Reset"=w1160, "Image Array In"=w1157, "Data Count"=w1161, "TCSPC Binning"=w1154) -> ("Image Array Out"=w1156:i32[][][])  [unwired: 2 in, 8 out]
                }
                n581 = Close File(refnum=w1133, error in=w1131) -> (error out=w1132:errorcluster)  [unwired: 1 out]
              }
            }
          }
          frame "Find Single Mol." {
            # "dirty trick"
            n582 = local read "Active pt3"() -> (w1205:path)
            n583 = call "MTS_GetFileFromWS.vi"(".pt3 File Name"=w1205) -> ("File Header"=w1204:T39)  [unwired: 9 in, 1 out]
            n584 = Unbundle By Name(w1204) -> ("Measurement Type"=w1203:T40, "Pixels"=w1191:i32[], "Upper Left"=w1200:T42, "Scan Axis"=w1199:enum32{"x-y", "x-z", "y-z"})
            n585 = local read "Picture size 2"() -> (w1186:dbl)
            n586 = local read "Picture size"() -> (w1189:dbl)
            n587 = local read "Resolution"() -> (w1187:dbl)
            n588 = local read "X-Position"() -> (w1180:dbl)
            n589 = local read "Y-Position"() -> (w1179:dbl)
            n590 = Divide(x=w1189, y=w1187) -> (x/y=w1188:dbl)
            n591 = Divide(x=w1186, y=w1187) -> (x/y=w1185:dbl)
            n592 = Equal?(x=T29."Image File" ("Measurement Type"), y=w1203) -> (x = y?=w1201:bool)
            n593 = call "MTS_ScannerXYZToImageXY.vi"("Axis"=w1199, "Scanner XYZ"=w1200) -> ("Image Y"=w1182:dbl, "Image X"=w1184:dbl)
            n594 = case shown="True" TRUE {
              tunnel: [w1208 w1211] -> w1190
              tunnel: w1191 -> [w1208 _]
              tunnel: w1188 -> [_ w1215]
              tunnel: w1185 -> [_ w1214]
              tunnel: [w1207 w1210] -> w1183
              tunnel: w1184 -> [w1207 _]
              tunnel: [w1206 w1209] -> w1181
              tunnel: w1182 -> [w1206 _]
              tunnel: w1180 -> [_ w1210]
              tunnel: w1179 -> [_ w1209]
              frame False {
              }
              frame True {
                n595 = To Long Integer(number=w1215) -> (32bit integer=w1213:i32)
                n596 = To Long Integer(number=w1214) -> (32bit integer=w1212:i32)
                n597 = Build Array(w1213, w1212) -> (w1211:i32[])
              }
            }
            n598 = Build Array(w1189, w1186) -> (w1195:dbl[])
            n599 = case shown="True" w1201 {
              tunnel: w1198 -> [w1216 w1291]
              tunnel: w1205 -> [_ _]
              tunnel: w1205 -> [_ _]
              tunnel: [w1216 w1296] -> w1196
              tunnel: w1190 -> [_ w1313]
              tunnel: w1195 -> [_ w1295]
              tunnel: w1183 -> [_ w1305]
              tunnel: w1181 -> [_ w1306]
              frame False {
              }
              frame True {
                w1265 = T11 1 items=["Center of Mass X", "Center of Mass Y", "First Pixel X", "First Pixel Y", "Bounding Rect Left", "Bounding Rect Top", "Bounding Rect Right", "Bounding Rect Bottom", "Max Feret Diameter Start X", "Max Feret Diameter Start Y", "Max Feret Diameter End X", "Max Feret Diameter End Y", "Max Horiz. Segment Length Left", "Max Horiz. Segment Length Right", "Max Horiz. Segment Length Row", "-", "Bounding Rect Width", "Bounding Rect Height", "Bounding Rect Diagonal", "Perimeter", "Convex Hull Perimeter", "Holes' Perimeter", "Max Feret Diameter", "Equivalent Ellipse Major Axis", "Equivalent Ellipse Minor Axis", "Equivalent Ellipse Minor Axis (Feret)", "Equivalent Rect Long Side", "Equivalent Rect Short Side", "Equivalent Rect Diagonal", "Equivalent Rect Short Side (Feret)", "Average Horiz. Segment Length", "Average Vert. Segment Length", "Hydraulic Radius", "Waddel Disk Diameter", "-", "Area", "Holes' Area", "Particle & Holes' Area", "Convex Hull Area", "Image Area", "-", "Number of Holes", "Number of Horiz. Segments", "Number of Vert. Segments", "-", "Orientation", "Max Feret Diameter Orientation", "-", "% Area/Image Area", "% Area/(Particle & Holes' Area)", "Ratio of Equivalent Ellipse Axes", "Ratio of Equivalent Rect Sides", "-", "Elongation Factor", "Compactness Factor", "Heywood Circularity Factor", "Type Factor", "-", "Sum X", "Sum Y", "Sum XX", "Sum XY", "Sum YY", "Sum XXX", "Sum XXY", "Sum XYY", "Sum YYY", "-", "Moment of Inertia XX", "Moment of Inertia XY", "Moment of Inertia YY", "Moment of Inertia XXX", "Moment of Inertia XXY", "Moment of Inertia XYY", "Moment of Inertia YYY", "Norm. Moment of Inertia XX", "Norm. Moment of Inertia XY", "Norm. Moment of Inertia YY", "Norm. Moment of Inertia XXX", "Norm. Moment of Inertia XXY", "Norm. Moment of Inertia XYY", "Norm. Moment of Inertia YYY", "Hu Moment 1", "Hu Moment 2", "Hu Moment 3", "Hu Moment 4", "Hu Moment 5", "Hu Moment 6", "Hu Moment 7"] ("Measurement Parameter")
                w1246 = TRUE ("Measurement Type")
                w1270 = T11 0 items=["Center of Mass X", "Center of Mass Y", "First Pixel X", "First Pixel Y", "Bounding Rect Left", "Bounding Rect Top", "Bounding Rect Right", "Bounding Rect Bottom", "Max Feret Diameter Start X", "Max Feret Diameter Start Y", "Max Feret Diameter End X", "Max Feret Diameter End Y", "Max Horiz. Segment Length Left", "Max Horiz. Segment Length Right", "Max Horiz. Segment Length Row", "-", "Bounding Rect Width", "Bounding Rect Height", "Bounding Rect Diagonal", "Perimeter", "Convex Hull Perimeter", "Holes' Perimeter", "Max Feret Diameter", "Equivalent Ellipse Major Axis", "Equivalent Ellipse Minor Axis", "Equivalent Ellipse Minor Axis (Feret)", "Equivalent Rect Long Side", "Equivalent Rect Short Side", "Equivalent Rect Diagonal", "Equivalent Rect Short Side (Feret)", "Average Horiz. Segment Length", "Average Vert. Segment Length", "Hydraulic Radius", "Waddel Disk Diameter", "-", "Area", "Holes' Area", "Particle & Holes' Area", "Convex Hull Area", "Image Area", "-", "Number of Holes", "Number of Horiz. Segments", "Number of Vert. Segments", "-", "Orientation", "Max Feret Diameter Orientation", "-", "% Area/Image Area", "% Area/(Particle & Holes' Area)", "Ratio of Equivalent Ellipse Axes", "Ratio of Equivalent Rect Sides", "-", "Elongation Factor", "Compactness Factor", "Heywood Circularity Factor", "Type Factor", "-", "Sum X", "Sum Y", "Sum XX", "Sum XY", "Sum YY", "Sum XXX", "Sum XXY", "Sum XYY", "Sum YYY", "-", "Moment of Inertia XX", "Moment of Inertia XY", "Moment of Inertia YY", "Moment of Inertia XXX", "Moment of Inertia XXY", "Moment of Inertia XYY", "Moment of Inertia YYY", "Norm. Moment of Inertia XX", "Norm. Moment of Inertia XY", "Norm. Moment of Inertia YY", "Norm. Moment of Inertia XXX", "Norm. Moment of Inertia XXY", "Norm. Moment of Inertia XYY", "Norm. Moment of Inertia YYY", "Hu Moment 1", "Hu Moment 2", "Hu Moment 3", "Hu Moment 4", "Hu Moment 5", "Hu Moment 6", "Hu Moment 7"] ("Measurement Parameter")
                w1285 = T43 4 items=["Grayscale (U8)", "Grayscale (I16)", "Grayscale (SGL)", "Complex (CSG)", "RGB (U32)", "HSL (U32)", "RGB (U64)", "Grayscale (U16)"] ("Image Type")
                w1293 = T43 4 items=["Grayscale (U8)", "Grayscale (I16)", "Grayscale (SGL)", "Complex (CSG)", "RGB (U32)", "HSL (U32)", "RGB (U64)", "Grayscale (U16)"] ("Image Type")
                w1312 = 1 ("index")
                # "Pixel Size [um]"
                n600 = Index Array(array=w1295, index #2=w1312) -> (element #1=w1311:dbl, element #2=w1308:dbl)  [unwired: 1 in]
                n601 = Index Array(array=w1313, index #2=w1312) -> (element #1=w1310:i32, element #2=w1309:i32)  [unwired: 1 in]
                n602 = Divide(x=w1311, y=w1310) -> (x/y=w1221:dbl)
                n603 = Divide(x=w1308, y=w1309) -> (x/y=w1307:dbl)
                n604 = Reciprocal(x=w1221) -> (1/x=w1222:dbl)
                n605 = Multiply(x=w1222, y="Focuswidth") -> (x*y=w1220:dbl)
                n606 = Random Number (0-1)() -> (number: 0 to 1=w1290:dbl)
                n607 = Number To Decimal String(number=w1290) -> (decimal integer string=w1289:string)  [unwired: 1 in]
                n608 = Concatenate Strings(w1289, "IMAQ CreatePatternimg" ("Image Name")) -> (w1287:string)
                n609 = call "IMAQ Create"("Image Name"=w1287, "Image Type"=w1293, "error in (no error)"=w1291) -> ("New Image"=w1292:T5, "error out"=w1280:errorcluster)  [unwired: 2 in]
                n610 = local read "Image"() -> (w1224:i32[][])
                n611 = call "MTS_IntensityArrayToImage.vi"(0:"Image"=w1292, 1:"Image"=w1224, "error in (no error)"=w1280, "Log Scale"=FALSE) -> ("Image Out"=w1245:T5, "error out"=w1237:errorcluster)  [unwired: 10 in]
                n612 = Random Number (0-1)() -> (number: 0 to 1=w1284:dbl)
                n613 = Array To Cluster(array=T32 [] ("MesaurementSelection")) -> (cluster=w1273:T44)
                n614 = Number To Decimal String(number=w1284) -> (decimal integer string=w1283:string)  [unwired: 1 in]
                n615 = Unbundle By Name(w1273) -> ("MesaurementSelection[0]"=w1271:T45, "MesaurementSelection[1]"=w1266:T45, "MesaurementSelection[2]"=w1261:T45, "MesaurementSelection[3]"=w1252:T45)
                n616 = Concatenate Strings(w1283, "IMAQ CreatePatternimg2" ("Image Name")) -> (w1281:string)
                n617 = call "IMAQ Create"("Image Name"=w1281, "Image Type"=w1285, "error in (no error)"=w1237) -> ("New Image"=w1279:T5, "error out"=w1236:errorcluster)  [unwired: 2 in]
                n618 = Bundle By Name(cluster=w1271, "Measurement Parameter"=w1270, "Range Lower Value"="X Start 2", "Range Upper Value"="X End 2", "Range"="Exclude / Include X", "Measurement Type"=w1246) -> (w1260:T45)
                n619 = Bundle By Name(cluster=w1266, "Measurement Parameter"=w1265, "Range Lower Value"="Y Start 2", "Range Upper Value"="Y End 2", "Range"="Exclude / Include Y", "Measurement Type"=w1246) -> (w1259:T45)
                n620 = Bundle By Name(cluster=w1261, "Measurement Parameter"="Measurement Parameter 1", "Range Lower Value"="Range Lower Value Par 1", "Range Upper Value"="Range Upper Value  Par 1", "Range"="Ex/In Par 1", "Measurement Type"=w1246) -> (w1258:T45)
                n621 = Bundle By Name(cluster=w1252, "Measurement Parameter"="Measurement Parameter 2", "Range Lower Value"="Range Lower Value Par 2", "Range Upper Value"="Range Upper Value Par 2", "Range"="Ex/In Par 2", "Measurement Type"=w1246) -> (w1251:T45)
                n622 = Build Array(w1260, w1259, w1258, w1251) -> (w1257:T32)
                n623 = call "MTS_IntensityArrayToImage.vi"(0:"Image"=w1279, 1:"Image"=w1224, "error in (no error)"=w1236, "Log Scale"=TRUE) -> ("Image Out"=w1230:T5, "error out"=w1235:errorcluster)  [unwired: 10 in]
                n624 = case shown="0, Default" "Detection Modus" {
                  tunnel: "Remove Outliers" -> [_ w1345]
                  tunnel: [w1322 w1336] -> w1286
                  tunnel: w1235 -> [w1327 w1344]
                  tunnel: [w1320 w1334] -> w1277
                  tunnel: "Filter" -> [_ w1343]
                  tunnel: w1257 -> [_ w1342]
                  tunnel: w1245 -> [_ w1337]
                  tunnel: path "C:/Users/Core-FCS/Desktop/Documents/AbelFCS/ParticleFinder/SingleMoleculePatternFinder/Patterns/azimutalGolden.png" ("Template File Path (GeometricMatching)") -> [_ _]
                  tunnel: "Settings (GeometricMatching)" -> [_ _]
                  tunnel: IMAQ_Rounding_Mode."Optimize" ("Rounding Mode Gaussian") -> [_ w1341]
                  tunnel: IMAQ_Rounding_Mode."Optimize" ("Rounding Mode Convolution") -> [_ w1340]
                  tunnel: "Square/Hexa" -> [_ w1339]
                  tunnel: "Connectivity 4/8" -> [_ w1338]
                  tunnel: w1230 -> [w1324 w1332]
                  tunnel: [w1324 w1329] -> w1234
                  tunnel: [w1326 w1330] -> w1232
                  tunnel: "Manual" -> [_ w1328]
                  tunnel: w1224 -> [w1318 _]
                  tunnel: "Mode" -> [w1317 _]
                  tunnel: w1220 -> [w1316 _]
                  tunnel: [w1315 _] -> w1218
                  tunnel: "NA" -> [w1314 _]
                  frame 0, Default {
                    n625 = To Double Precision Float(number=w1318) -> (double precision float=w1319:dbl[][])
                    n626 = script code="addpath(path);\nswitch (mode)\ncase 0\nmaskGauss = GenGauss2D(focus);\n[err,bim,cim,sim,yc,xc,bc,cc,sc,len,imm]=FindPatternCP(image,maskGauss,[],[],[],1.5);\npattern=maskGauss;\ncase 1\nmaskRad=Radialpattern_gen('radial', focus,NA);\n[err,bim,cim,sim,yc,xc,bc,cc,sc,len,imm]=FindPatternCP(image,maskRad,[],[],[],1);\npattern=maskRad(:,:,15);\ncase 2\nmaskAzi=Radialpattern_gen('azimuthal', focus,NA);\n[err,bim,cim,sim,yc,xc,bc,cc,sc,len,imm]=FindPatternCP(image,maskAzi,[],[],[],1.5);\npattern=maskAzi(:,:,15);\nend\nxc=xc-1;\nyc=yc-1;"("??"=w1327, "path"="C:\\Users\\Core-FCS\\Desktop\\Documents\\CoreSetupNew\\MatlabLibAbelFCS", "image"=w1319, "mode"=w1317, "focus"=w1316, "NA"=w1314) -> ("??"=w1326:errorcluster, "pattern"=w1315:dbl[][], "xc"=w1323:dbl[], "yc"=w1321:dbl[])
                    n627 = Build Array(w1323, w1321) -> (w1322:dbl[][])
                    n628 = Array Size(array=w1321) -> (size(s)=w1320:i32)
                  }
                  frame 1 {
                    n629 = call "SingleMoleFinderEasy.vi"("Image Src"=w1337, "Number of Erosion"=w1345, "HolesBorder"=w1343, "Selection Values"=w1342, "Rounding Mode Gaussian"=w1341, "error in"=w1344, "Rounding Mode Convolution"=w1340, "Square/Hexa (Square)"=w1339, "Connectivity 4/8 (8)"=w1338) -> ("Number of Particles"=w1333:i32, "Particle Measurements (Pixels)"=w1335:dbl[][], "error out"=w1331:errorcluster)  [unwired: 15 in, 1 out]
                    n630 = case shown="True" w1328 {
                      tunnel: w1331 -> [w1349 w1357]
                      tunnel: [w1349 w1356] -> w1330
                      tunnel: [w1346 w1355] -> w1329
                      tunnel: [w1347 w1354] -> w1336
                      tunnel: w1335 -> [w1347 w1351]
                      tunnel: [w1348 w1353] -> w1334
                      tunnel: w1333 -> [w1348 w1352]
                      tunnel: w1332 -> [w1346 w1350]
                      frame False {
                      }
                      frame True {
                        n631 = while {
                          tunnel: w1357 -> [w1372]
                          tunnel: [w1371] -> w1356
                          tunnel: w1350 -> [w1370]
                          tunnel: [w1369] -> w1355
                          shift-right: [w1362] -> w1354
                          shift-left: w1351 -> [w1361]
                          tunnel: [w1360] -> w1353
                          tunnel: w1352 -> [w1359]
                          i -> [w1366]
                          stop <- w1368 stop-if-true
                          n632 = call "IMAQ Select Point"("Window Number (0...15)"=1, "error in (no error)"=w1372, "Image In"=w1370) -> ("error out"=w1371:errorcluster, "Cancelled"=w1368:bool, "Point"=w1367:T46, "Image Out (duplicate)"=w1369:T5)  [unwired: 5 in]
                          n633 = Unbundle(w1367) -> ("X"=w1365:sgl, "Y"=w1364:sgl)
                          n634 = Build Array(w1365, w1364) -> (w1363:sgl[])
                          n635 = Add(x=w1359, y=w1366) -> (x+y=w1360:i32)
                          n636 = Insert Into Array(array=w1361, index (row)=w1360, new element=w1363) -> (w1362:dbl[][])  [unwired: 1 in]
                        }
                      }
                    }
                  }
                }
                "Number of Particles" <- w1277
                "Image 2" <- w1218
                n637 = Index Array(array=w1286, index (col) #1=0 ("index (row)"), index (col) #2=1 ("index (col)")) -> (element #1=w1229:dbl[], element #2=w1227:dbl[])  [unwired: 2 in]
                n638 = Multiply(x=w1221, y=w1229) -> (x*y=w1304:dbl[])
                n639 = Multiply(x=w1227, y=w1307) -> (x*y=w1303:dbl[])
                n640 = To Word Integer(number=w1229) -> (16bit integer=w1228:i16[])
                n641 = To Word Integer(number=w1227) -> (16bit integer=w1226:i16[])
                n642 = Add(x=w1305, y=w1304) -> (x+y=w1299:dbl[])
                n643 = Add(x=w1303, y=w1306) -> (x+y=w1298:dbl[])
                n644 = for {
                  N: w1277 -> [_]
                  shift-right: [w1379] -> w1233
                  shift-left: w1234 -> [w1380]
                  tunnel: w1228 -> [w1378] mode=indexing
                  tunnel: w1226 -> [w1377] mode=indexing
                  shift-right: [w1381] -> w1231
                  shift-left: w1232 -> [w1382]
                  tunnel: u32 16738560 -> [w1376]
                  tunnel: 3.0 ("x") -> [w1375]
                  n645 = call "MTS_DrawCrossIMAQIamge.vi"("Image"=w1380, "Size"=w1375, "Color"=w1376, "X"=w1378, "Y"=w1377, "error in (no error)"=w1382) -> ("Image Out"=w1379:T5, "error out"=w1381:errorcluster)  [unwired: 8 in]
                }
                "AM image" <- w1233
                n646 = Build Array(w1299, w1298, w1228, w1226) -> (→"Pattern":dbl[][])
                n647 = global write "patternImg.vi" "New Image"(w1233) -> ()
                n648 = flat-sequence {
                  tunnel: w1231 -> [w1374]
                  tunnel: [w1374] -> w1296
                  frame #0 {
                    n649 = local write "Tab Control"(T4."AutoMesaurement" ("Tab Control")) -> ()
                  }
                }
              }
            }
          }
          frame "Auto Measurement Control" {
            # "Init"
            n650 = local read "Pattern"() -> (w1393:dbl[][])
            n651 = Index Array(array=w1393, index (row) #1=2 ("index (row)"), index (row) #2=3 ("index (col)")) -> (element #1=w1390:dbl[], element #2=→"subarray":dbl[])  [unwired: 2 in]
            n652 = local read "NxtAutMesPoint"() -> (w1401:i32)
            n653 = Array Size(array=w1390) -> (size(s)=w1389:i32)
            n654 = Less Than 0?(x=w1401) -> (x < 0?=w1404:bool)
            n655 = case shown="False" w1404 {
              tunnel: w1398 -> [w1425 w1429]
              tunnel: [w1425 w1428] -> w1402
              tunnel: [w1424 w1426] -> w1400
              tunnel: w1389 -> [_ w1426]
              frame False {
                n656 = local read "Auto Measure Points"() -> (w1424:i32)
              }
              frame True {
                n657 = Number To Decimal String(number=w1426) -> (decimal integer string=w1431:string)  [unwired: 1 in]
                n658 = Concatenate Strings("Point 1 / " ("Caption.Text"), w1431) -> (w1430:string)
                n659 = property on="Auto Meas Progress" class="Slide (strict)"(error in=w1429, "Scale.Minimum"=0.0 ("Scale.Range:Minimum"), "Scale.Maximum"=w1426, "Value"=1 ("Auto Meas Progress"), "Caption.Text"=w1430) -> (error out=w1428:errorcluster)  [unwired: 1 in, 1 out]
                "Auto Measure Points" <- w1426
              }
            }
            n660 = Increment(x=w1401) -> (x+1=w1384:i32)
            "NxtAutMesPoint" <- w1384
            n661 = Greater Or Equal?(x=w1384, y=w1400) -> (x >= y?=w1403:bool)
            n662 = Increment(x=w1384) -> (x+1=w1399:i32)
            n663 = Index Array(array=w1393, index (row) #1=2 ("index (row)"), index (col) #1=w1384, index (row) #2=3 ("index (col)"), index (col) #2=w1384) -> (element #1=w1392:dbl, element #2=w1391:dbl)
            n664 = case shown="False" w1403 {
              tunnel: w1402 -> [w1415 w1423]
              tunnel: [w1421 w1423] -> w1396
              tunnel: [T14."Auto Point" ("Do Measurement") T14."No Measurement" ("Do Measurement")] -> w1395
              tunnel: w1399 -> [w1416 _]
              tunnel: w1392 -> [w1413 _]
              tunnel: w1391 -> [w1412 _]
              tunnel: w1400 -> [w1409 _]
              frame False {
                # "Prpare For Next Point"
                # "1 loc max  2 undef 0 saddle -1 local min"
                n665 = global read "patternImg.vi" "New Image"() -> (w1405:T5)
                n666 = Number To Decimal String(number=w1416) -> (decimal integer string=w1418:string)  [unwired: 1 in]
                n667 = Number To Decimal String(number=w1409) -> (decimal integer string=w1410:string)  [unwired: 1 in]
                n668 = Concatenate Strings("Point " ("Caption.Text"), w1418, " / " ("Caption.Text"), w1410) -> (w1417:string)
                n669 = call "MTS_DrawCrossIMAQIamge.vi"("Image"=w1405, "Size"=3.0 ("x"), "Color"=u32 6618880, "X"=w1413, "Y"=w1412, "error in (no error)"=w1415) -> ("Image Out"=w1406:T5, "error out"=w1414:errorcluster)  [unwired: 8 in]
                n670 = local write "AM image"(w1406) -> ()
                n671 = property on="Auto Meas Progress" class="Slide (strict)"(error in=w1414, "Value"=w1416, "Caption.Text"=w1417) -> (error out=w1421:errorcluster)  [unwired: 1 in, 1 out]
              }
              frame True {
                # "No More Points"
              }
            }
          }
        }
        n672 = local write "Buffer Overrun"(w573) -> ()
      }
      frame Error {
      }
    }
    n673 = Unbundle(w558) -> ("status"=w557:bool)  [unwired: 2 out]
    n674 = flat-sequence {
      tunnel: w561 -> [w1449]
      tunnel: [w1449] -> w560
      tunnel: w556 -> [w1446]
      frame #0 {
        n675 = local write "Task"(w1446) -> ()
        n676 = Equal?(x=w1446, y=T25."No Measurement" ("Do Measurement")) -> (x = y?=w1447:bool)
        n677 = Not(x=w1447) -> (.not. x?=w1448:bool)
        n678 = local write "Running"(w1448) -> ()
      }
    }
    n679 = local read "Global Stop"() -> (w564:bool)
    n680 = Compound Arithmetic op=OR(w557, w562, w564) -> (w563:bool)
  }
  n681 = while {
    tunnel: w6 -> [w1450]
    tunnel: [w1451] -> _
    stop <- w1454 stop-if-true
    n682 = property on="3dAbelFcs" class="Bool (strict)"(error in=w1450) -> (error out=w1452:errorcluster, "Value"=w1453:bool)  [unwired: 1 in, 1 out]
    n683 = local read "Global Stop"() -> (w1454:bool)
    n684 = case shown="False" w1453 {
      tunnel: w1452 -> [_ w1463]
      tunnel: [_ w1469] -> w1451
      frame False {
      }
      frame True {
        n685 = local read "Z Stepsize"() -> (w1466:dbl)
        n686 = local read "Y Stepsize"() -> (w1467:dbl)
        n687 = local read "X Stepsize"() -> (w1468:dbl)
        n688 = local read "Z Steps"() -> (w1465:dbl)
        n689 = call "SetShutter.vi"("type"=Shutter_type_typedef."TTL High", "mode"=Shutter_mode_typedef."Open", "error in (no error)"=w1463) -> ("error out"=w1455:errorcluster)  [unwired: 11 in, 1 out]
        n690 = for {
          N: w1465 -> [_]
          tunnel: w1455 -> [w1479]
          tunnel: w1466 -> [w1484]
          tunnel: w1467 -> [w1483]
          tunnel: w1468 -> [w1482]
          tunnel: [w1478] -> w1464
          tunnel: w1465 -> [w1477]
          i -> [w1481]
          n691 = local read "Z Start"() -> (w1471:dbl)
          n692 = local write "Z-Position"(w1471) -> ()
          n693 = Multiply(x=w1484, y=w1481) -> (x*y=w1475:dbl)
          n694 = Subtract(x=200, y=w1471) -> (x-y=w1472:dbl)
          n695 = local read "Y Steps"() -> (w1476:dbl)
          n696 = Add(x=w1472, y=w1475) -> (x+y=w1473:dbl)
          n697 = Number To Decimal String(number=w1481) -> (decimal integer string=w1480:string)  [unwired: 1 in]
          n698 = for {
            N: w1476 -> [_]
            tunnel: w1483 -> [w1522]
            tunnel: w1482 -> [w1521]
            tunnel: w1479 -> [w1518]
            tunnel: w1480 -> [w1520]
            tunnel: [w1492] -> w1478
            tunnel: w1471 -> [w1489]
            tunnel: w1477 -> [w1513]
            tunnel: w1476 -> [w1512]
            tunnel: w1473 -> [w1510]
            i -> [w1494]
            w1490 = "_" ("string")
            n699 = local read "X Steps"() -> (w1511:dbl)
            n700 = Number To Decimal String(number=w1494) -> (decimal integer string=w1519:string)  [unwired: 1 in]
            n701 = for {
              N: w1511 -> [_]
              tunnel: w1518 -> [w1537]
              tunnel: w1521 -> [w1542]
              tunnel: [w1538] -> w1516
              tunnel: w1520 -> [w1540]
              tunnel: w1519 -> [w1539]
              shift-right: [w1536] -> w1515
              shift-left: _ -> [w1535]
              tunnel: [w1534] -> w1514
              tunnel: [w1532] -> w1509
              tunnel: [w1533] -> w1508
              i -> [w1541]
              n702 = control-ref of="Stop Measurement"() -> (w1528:refnum<vi>)
              n703 = control-ref of="Point Measurement"() -> (w1523:refnum<vi>)
              n704 = control-ref of="Running"() -> (w1531:refnum<vi>)
              n705 = control-ref of="FCS Point Measurement"() -> (w1526:refnum<vi>)
              n706 = control-ref of="concatenated string"() -> (w1524:refnum<vi>)
              n707 = control-ref of="Workspace"() -> (w1529:refnum<vi>)
              n708 = control-ref of="X-Position"() -> (w1527:refnum<vi>)
              n709 = control-ref of="X Start"() -> (w1525:refnum<vi>)
              n710 = control-ref of="Task"() -> (w1530:refnum<vi>)
              n711 = call "LifeTimeImagePoint.vi"("Boolean in"=w1531, "String"=w1539, "reference 6"=w1527, "String 2"=w1540, "reference 7"=w1526, "error in (no error)"=w1537, "reference 4"=w1528, "reference 3"=w1529, "reference 9"=w1525, "reference in"=w1530, "Numeric in"=w1541, "Str Refnum"=w1524, "X Stepsize"=w1542, "Array in"=w1535, "Point Measurement"=w1523) -> ("Array out"=w1536:i32[][], "CCD Chip Size"=w1533:i32, "X Start"=w1534:dbl, "Numeric out"=w1532:dbl, "error out"=w1538:errorcluster)  [unwired: 8 in]
            }
            n712 = property on="Workspace" class="Path"() -> ("Value"=w1491:path)  [unwired: 2 in, 2 out]
            n713 = Increment(x=w1494) -> (x+1=w1495:i32)
            n714 = Get Date/Time In Seconds() -> (seconds since 1Jan1904=w1500:timestamp)
            n715 = Strip Path(path=w1491) -> (stripped path=w1504:path)  [unwired: 1 out]
            n716 = Format Date/Time String(time format string (%c)="%d%m%y_%H%M", seconds (now)=w1500) -> (date/time string=w1498:string)  [unwired: 1 in]
            n717 = Path To String(path=w1504) -> (string=w1505:string)
            n718 = Number To Decimal String(number=w1495) -> (decimal integer string=w1501:string)  [unwired: 1 in]
            n719 = local read "Y Start"() -> (w1485:dbl)
            n720 = local write "Y-Position"(w1485) -> ()
            n721 = Concatenate Strings(w1505, "\\" ("string"), "AreaISM" ("string"), w1490, w1501, w1490, w1498, w1490, w1490) -> (w1506:string)
            n722 = Multiply(x=w1522, y=w1494) -> (x*y=w1517:dbl)
            n723 = Subtract(x=200, y=w1485) -> (x-y=w1486:dbl)
            n724 = Add(x=w1486, y=w1517) -> (x+y=w1487:dbl)
            n725 = String To Path(string=w1506) -> (path=w1497:path)
            n726 = Build Array(w1489, w1485, w1514, w1513, w1512, w1511, w1510, w1487, w1509, w1508) -> (w1507:dbl[])
            n727 = Path To String(path=w1497) -> (string=w1496:string)
            n728 = script code="results.ImagePlane=Data;\nresults.Info.Zstart=Meta(1);\nresults.Info.Ystart=Meta(2);\nresults.Info.Xstart=Meta(3);\nresults.Info.Zsteps=Meta(4);\nresults.Info.Ysteps=Meta(5);\nresults.Info.Xsteps=Meta(6);\nresults.Info.Zpos=Meta(7);\nresults.Info.Ypos=Meta(8);\nresults.Info.Xpos=Meta(9);\nresults.Info.CcdSize=Meta(13);\nsave(file,'results');\nclear results;"("??"=w1516, "Data"=w1515, "Meta"=w1507, "file"=w1496) -> ("??"=w1493:errorcluster)
            n729 = call "FreeInternalMemory.vi"("error in (no error)"=w1493) -> ("error out"=w1492:errorcluster)  [unwired: 1 in, 1 out]
          }
        }
        n730 = call "AbortAcquisition.vi"("error in (no error)"=w1464) -> ("error out"=w1461:errorcluster)  [unwired: 1 in, 1 out]
        n731 = call "SetShutter.vi"("type"=Shutter_type_typedef."TTL High", "mode"=Shutter_mode_typedef."Close", "error in (no error)"=w1461) -> ("error out"=w1457:errorcluster)  [unwired: 11 in, 1 out]
        n732 = call <vilib>:"Clear Errors.vi"("error in (no error)"=w1457) -> ("error out"=w1456:errorcluster)  [unwired: 6 in]
        n733 = property on="3dAbelFcs" class="Bool (strict)"(error in=w1456, "Value"=FALSE ("3dAbelFcs")) -> (error out=w1469:errorcluster)  [unwired: 1 in, 1 out]
      }
    }
  }
  n734 = call "PulseTrain.vi"("error in"=w6, "duty cycle"="duty cycle", "frequency"="frequency") -> ("error out"=w5:errorcluster, "task out"=w4:refnum<k21>)  [unwired: 7 in]
  n735 = while {
    tunnel: [w1543] -> w7
    tunnel: w5 -> [w1543]
    tunnel: w4 -> [w1544]
    tunnel: [w1544] -> w3
    stop <- w1546 stop-if-true
    n736 = Wait (ms)(milliseconds to wait=u32 100) -> ()  [unwired: 1 out]
    n737 = local read "Global Stop"() -> (w1546:bool)
  }
  n738 = call <vilib>:"DAQmx Clear Task.vi"("task in"=w3, "error in"=w7) -> ()  [unwired: 13 in, 1 out]
  n739 = global read "patternImg.vi" "New Image"() -> (w8:T5)
  n740 = call "IMAQ Dispose"("Image"=w8, "error in (no error)"=w10) -> ()  [unwired: 4 in, 1 out]
